vi "EC_Applied_Motion_RXRYRZ_20120124_3ch.vi"() -> ()   [LabVIEW 2014]
uses:
  <vilib>/Utility/file.llb/Read From Spreadsheet File (I64).vi
  <vilib>/Utility/file.llb/Read From Spreadsheet File (string).vi
  <vilib>/Instr/_visa.llb/VISA Configure Serial Port (Instr).vi
  <userlib>/caLab/Private/Put_DBL-1D_PV-1D.vi
  <vilib>/Utility/file.llb/Write To Spreadsheet File (I64).vi
  <vilib>/Utility/file.llb/Write To Spreadsheet File (string).vi
panel:
  out "Z Velocity MV mm/sec":dbl format="%.3f"
  out "Z Position MV mm":dbl
  out "Y Velocity MV mm/sec":dbl format="%.3f"
  out "Y Position MV mm":dbl
  out "X Velocity MV mm/sec":dbl format="%.3f"
  out "X Position MV mm":dbl
  out "Presets":i32[][](array[numeric])
  in  "stop":bool
  in  "Tab Control 3":enum32{"Status", "Reset"}(tab)
  out "Y in Range":bool
  out "Y Scan":bool
  out "Y in Motion":bool
  out "Y Backlash corr":bool
  out "X  in Range":bool
  out "X Scan":bool
  out "X  in Motion":bool
  out "X Backlash corr":bool
  out "Z in Range":bool
  out "Z Scan":bool
  out "Z in Motion":bool
  out "Z Backlash corr":bool
  out "X Ready":bool
  out "Y Ready":bool
  out "Z Ready":bool
  in  "Reset Y Position mm":dbl
  out "Reset Y Motor Steps":i32
  in  "Reset X Position mm":dbl
  out "Reset X Motor Steps":i32
  in  "Reset Z Position mm":dbl
  out "Reset Z Motor Steps":i32
  in  "Reset":bool
  in  "Tab Control 2":enum32{"mm", "step"}(tab)
  in  "X Scan Length SP mm":dbl
  in  "X Scan Velocity SP mm/sec":dbl
  in  "X Scan set":bool
  in  "Y Scan Length SP mm":dbl
  in  "Y Scan Velocity SP mm/sec":dbl
  in  "Y Scan set":bool
  in  "Z Scan Length SP mm":dbl
  in  "Z Scan Velocity SP mm/sec":dbl
  in  "Z Scan set":bool
  in  "X Scan Velocity SP steps/sec":i32=1 min=1 max=102400 step=1
  in  "X Scan Length SP steps":i32 min=-500000 max=500000 step=100
  out "X Scan length MV mm":dbl
  out "X Scan velocity MV mm/sec":dbl format="%#_6f"
  in  "Y Scan Velocity SP steps/sec":i32=1 min=1 max=102400 step=1
  in  "Y Scan Length SP steps":i32 min=-1000000 max=0 step=100
  out "Y Scan length MV mm":dbl
  out "Y Scan velocity MV mm/sec":dbl format="%#_6f"
  in  "Z Scan Velocity SP steps/sec":i32=1 min=1 max=102400 step=1
  in  "Z Scan Length SP steps":i32 min=-204724 max=102195276 step=100
  out "Z Scan length MV mm":dbl
  out "Z Scan velocity MV mm/sec":dbl format="%#_6f"
  out "atan Y/Z":dbl
  in  "Tab Control":enum32{"mm", "preset", "step"}(tab)
  in  "X Position SP mm":dbl
  in  "X Velocity SP mm/sec":dbl
  in  "X Move Set":bool
  in  "Y Move Set":bool
  in  "Y Position SP mm":dbl
  in  "Y Velocity SP mm/sec":dbl
  in  "Z Position SP mm":dbl
  in  "Z Velocity SP mm/sec":dbl
  in  "Z Move Set":bool
  in  "Add Button":bool
  in  "String":string
  in  "Delete Button":bool
  in  "Preset positions":i32(ring) items=["ZERO", "Default", "CDOSE", "QMS", "test", "test2", "test3"]
  in  "Set Button":bool
  in  "X Velocity SP step/sec":i32 min=1 max=50000
  in  "Y Velocity SP step/sec":i32 min=1 max=50000
  in  "Z Velocity SP step/sec":i32 min=1 max=5000
  in  "Y Step SP":i32=-20000 min=-800000 max=800000 step=500
  in  "X Step SP":i32=-20000 min=-750000 max=750000 step=500
  in  "Z Step SP":i32=-20000 min=-3000 max=102400000 step=500
  out "X Step PV":i32 max=2000
  out "Y Step PV":i32 max=2000
  out "Z Step PV":i32 max=2000
  out "R Step PV":i32 max=2000
  out "X Scan Duration":dbl
  out "Y Scan Duration":dbl
  out "Z Scan Duration":dbl
  out "Z COM PORT":refnum<visa-resource-name>="COM5"
  out "Z Backlash steps/sec":i32
  out "Z Backlash":i32
  out "Z Holding Current %":i32
  out "Z Run Current %":i32
  out "Z offset mm":dbl
  out "Z mm/rev":dbl
  out "Z steps/rev":u32
  out "Z  velocity PV step/sec":i32
  out "Z MINPOS":i32=-94296
  out "Z MAXPOS":i32=-34296
  in  "Z Scan OK":bool
  in  "Z Go":bool
  out "Z Position mm PV":dbl
  out "X Position mm PV":dbl
  out "X velocity PV step/sec":i32
  in  "X Scan OK":bool
  in  "X Go":bool
  out "X Backlash steps/sec":i32
  out "X Backlash":i32
  out "X Holding Current %":i32
  out "X Run Current %":i32
  out "X offset mm":dbl
  out "X mm/rev":dbl
  out "X steps/rev":u32
  out "X MAXPOS":i32=-34296
  out "X MINPOS":i32=-94296
  out "X COM PORT":refnum<visa-resource-name>="COM5"
  out "Y Backlash steps/sec":i32
  out "Y Backlash":i32
  out "Y Holding Current %":i32
  out "Y Run Current %":i32
  in  "Scan Cancel":bool
  out "Y Position mm PV":dbl
  out "Y offset mm":dbl
  out "Y mm/rev":dbl
  out "Y steps/rev":u32
  out "Y velocity PV step/sec":i32
  in  "Y Scan OK":bool
  in  "Scan Go":bool
  in  "Stop":bool
  in  "Y Go":bool
  out "Y MINPOS":i32=-94296
  out "Y MAXPOS":i32=-34296
  out "Y COM PORT":refnum<visa-resource-name>="COM5"
  # "REF"
  # "Current position"
  # "Goto position"
  # "RX"
  # "RX"
  # "RY"
  # "RY"
  # "RZ"
  # "RZ"
  # "21-22-23"
  # "R,L = green"
  # "COM21:COM22:COM23"
  # "L"
  # "M"
  # "B"
  # "S"
  # "R"
  # "Preset position"
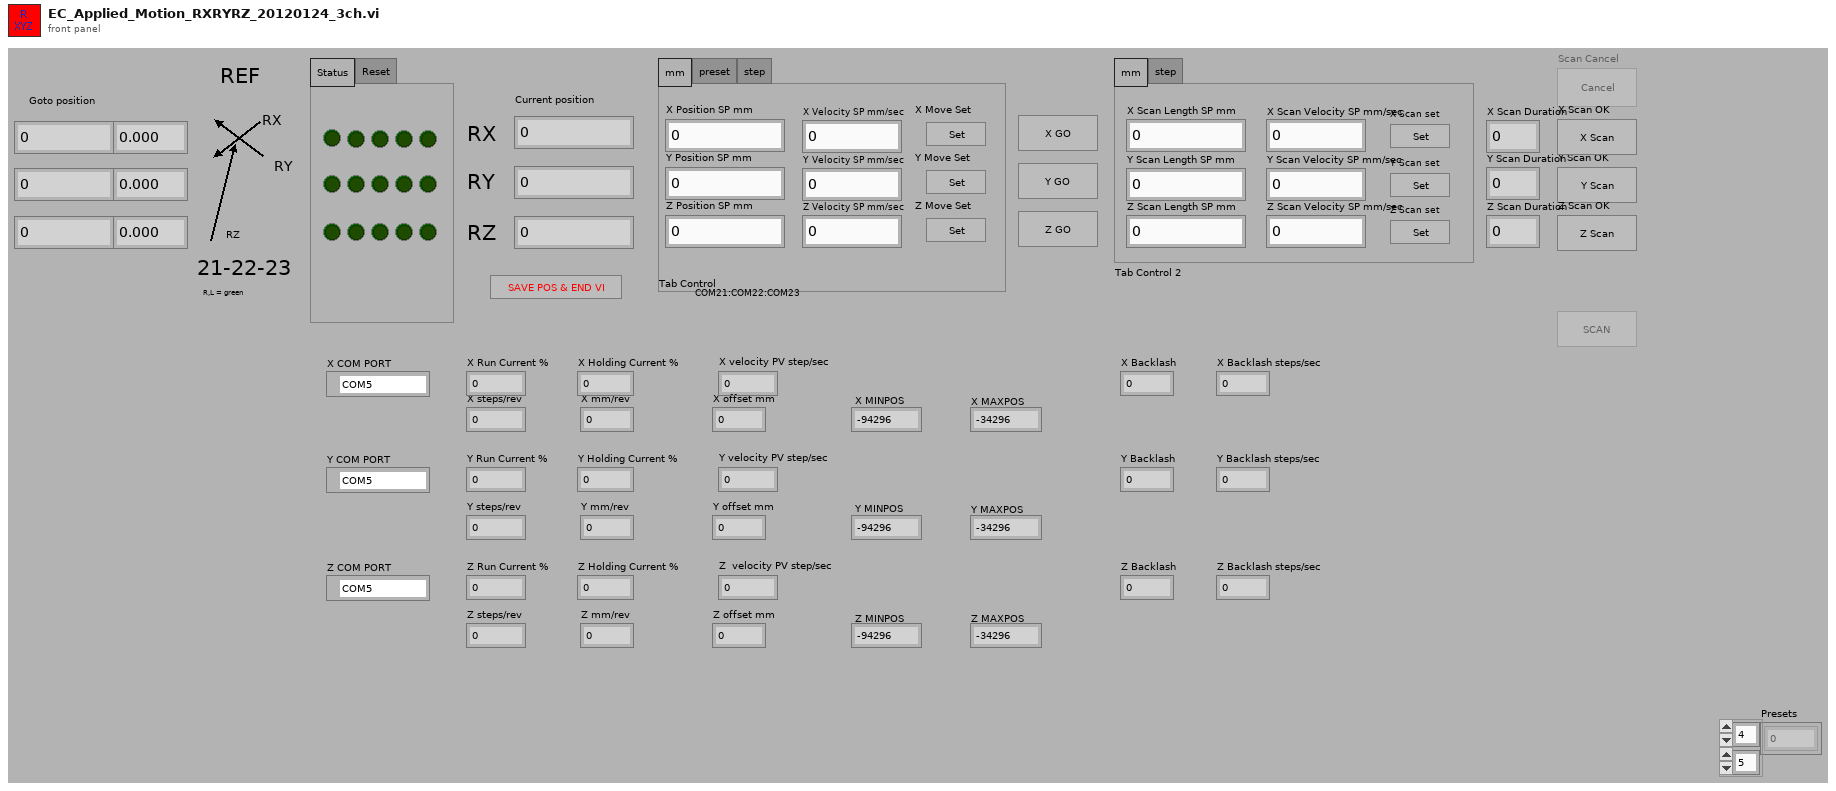
[diagram p1: front panel]
types:
  T1 = enum16{"Power-up Signature", "Accel Rate", "Accel Max", "Bit Rate", "Buffer Status", "Change Current", "Commence Jogging", "Change Jog Speed", "Continue", "Define Address", "Distance for FC,FM,FO,FY", "Decel Rate", "Distance or Position", "Define Limits", "Encoder Deadband", "Encoder Function", "Encoder Position", "Encoder Ratio", "Feed to Length with Speed Change", "Feed to Length", "Feed to Sensor with Mask Dist", "Feed to Length & Set Output", "Feed to Position", "Feed to Sensor", "Feed to Sensor w/safety", "Follow Handwheel", "Immediate Distance?", "Immediate Encoder?", "Immediate Low Output", "Immediate High Output", "Immediate Position?", "Input Status?", "Jog Accel/Decel", "Jog Disable", "Jog Enable", "Jog Speed", "Motor Disable", "Motor Enable", "Microstep Resolution", "Power up Current", "Power up Mode", "Pause", "Request Status", "Revision Level?", "Seek Home", "Stop Jogging", "Stop & Kill Buffer", "Set Output", "Set ABS Position", "Send String", "Stop", "Velocity for Speed Change", "Velocity Setting", "Wait for Input", "Wait Time"}
  T2 = enum8{"Enabled", "Disabled", "Disabled and Grayed Out"}
  T3 = cluster{"first row[0]":i64, "first row[1]":i64, "first row[2]":i64, "first row[3]":i64, "first row[4]":i64, "first row[5]":i64, "first row[6]":i64, "first row[7]":i64, "first row[8]":i64}
  T4 = cluster{"Value[0]":i32, "Value[1]":i32, "Value[2]":i32, "Value[3]":i32, "Value[4]":i32, "Value[5]":i32, "Value[6]":i32, "Value[7]":i32, "Value[8]":i32}
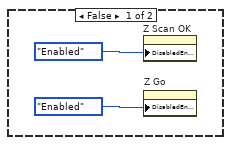
[diagram p5: hidden frame]
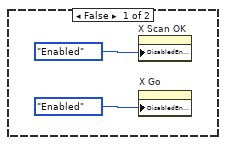
[diagram p8: hidden frame]
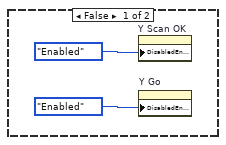
[diagram p11: hidden frame]
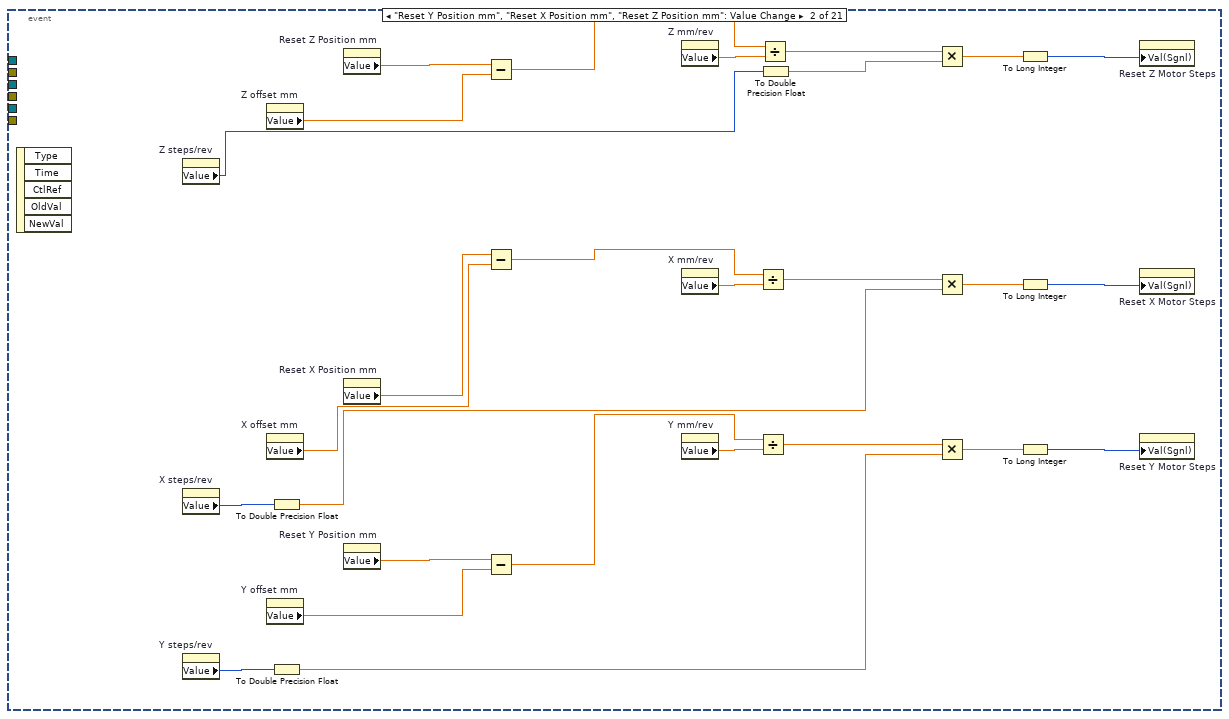
[diagram p14: hidden frame]
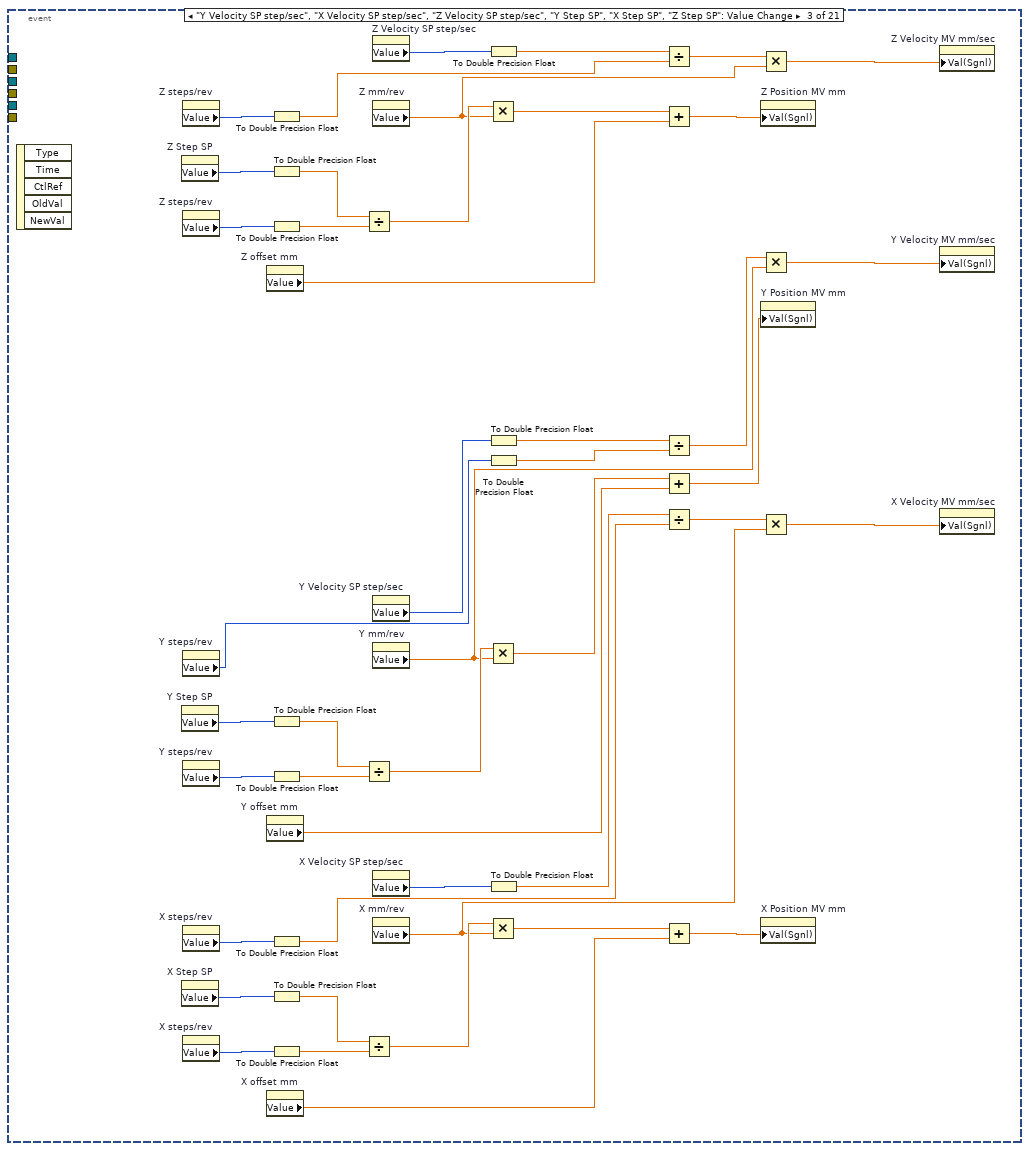
[diagram p15: hidden frame]
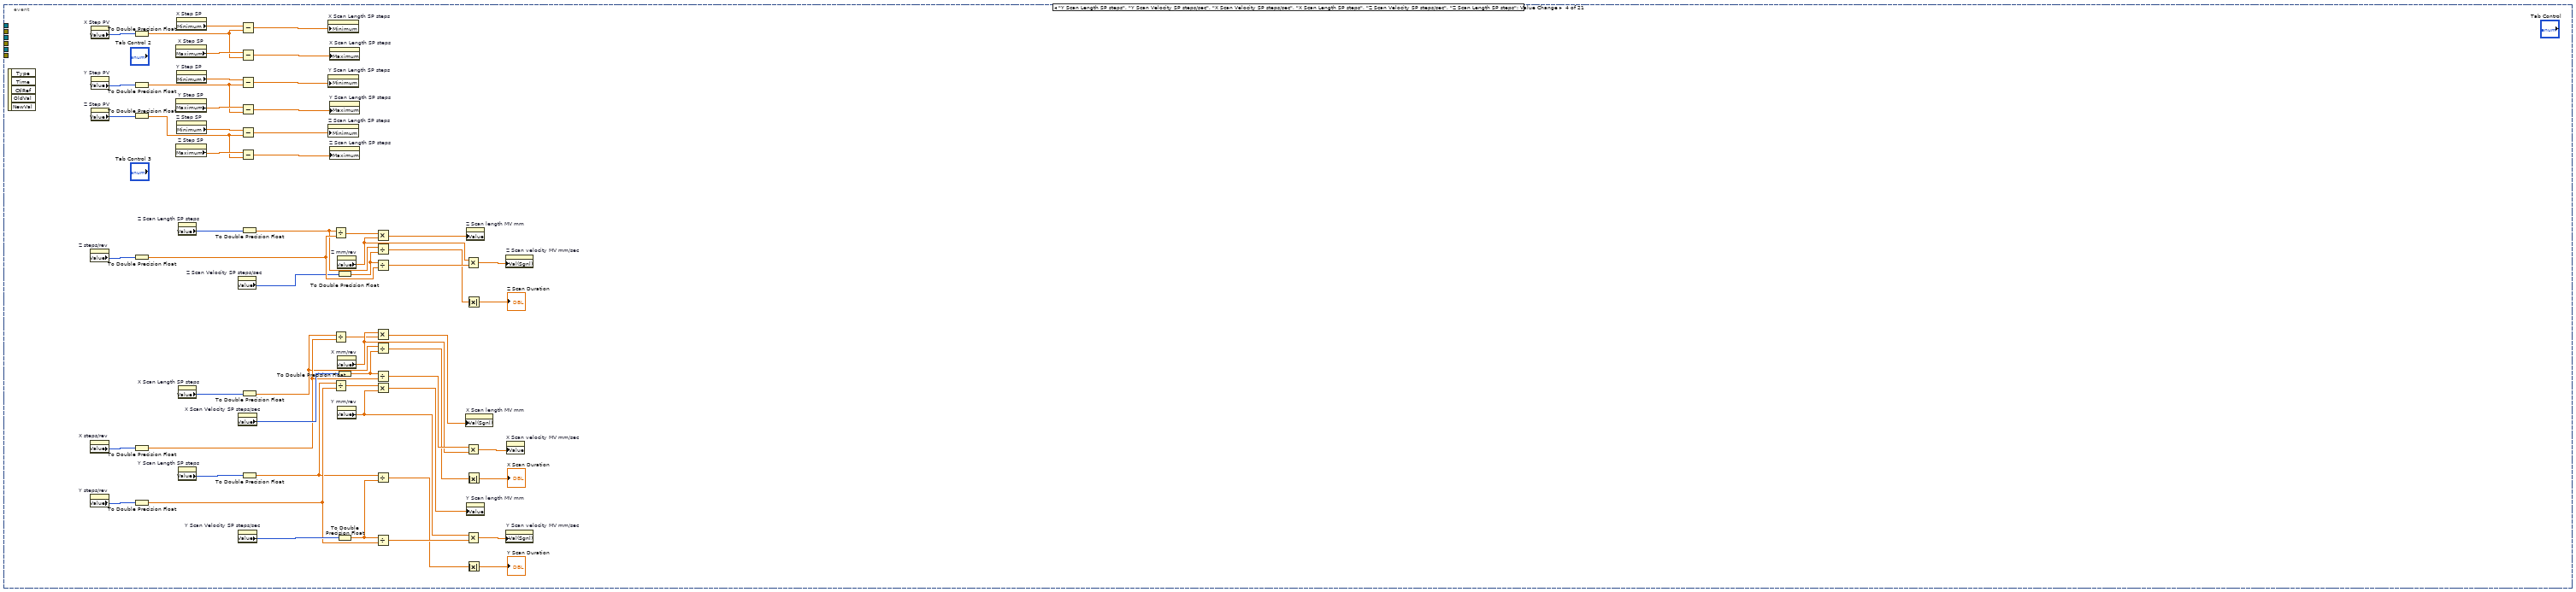
[diagram p16: hidden frame]
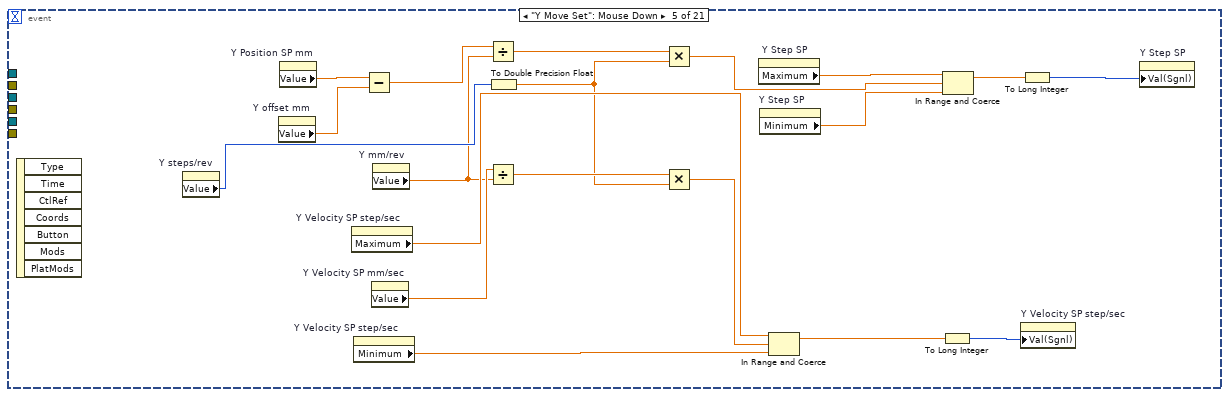
[diagram p17: hidden frame]
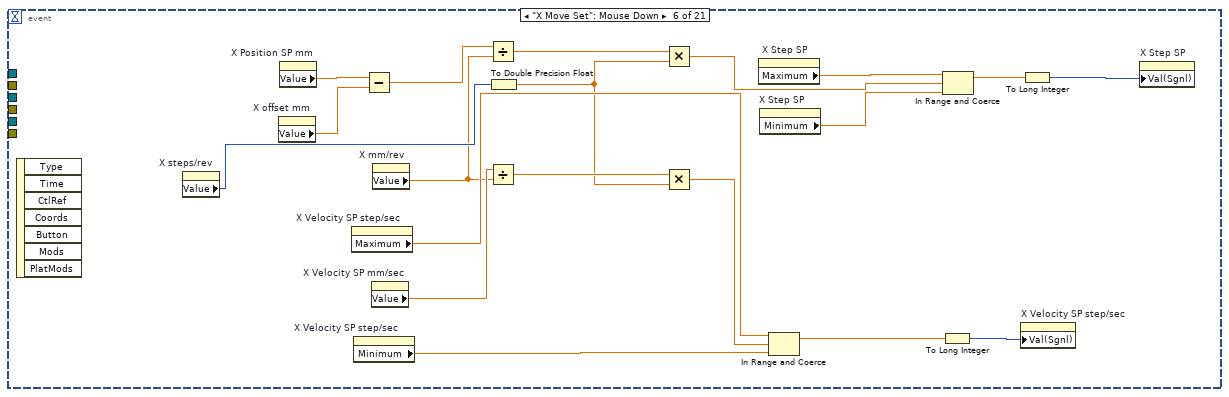
[diagram p18: hidden frame]
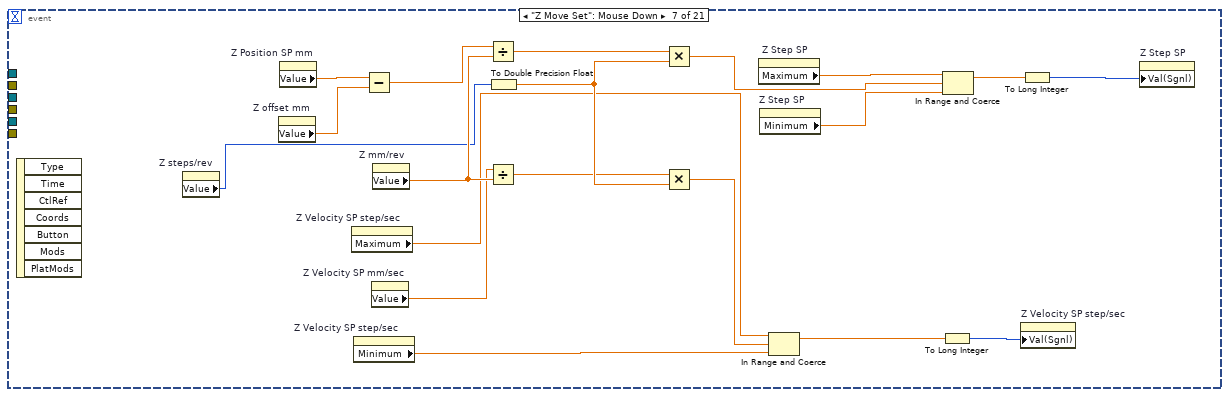
[diagram p19: hidden frame]
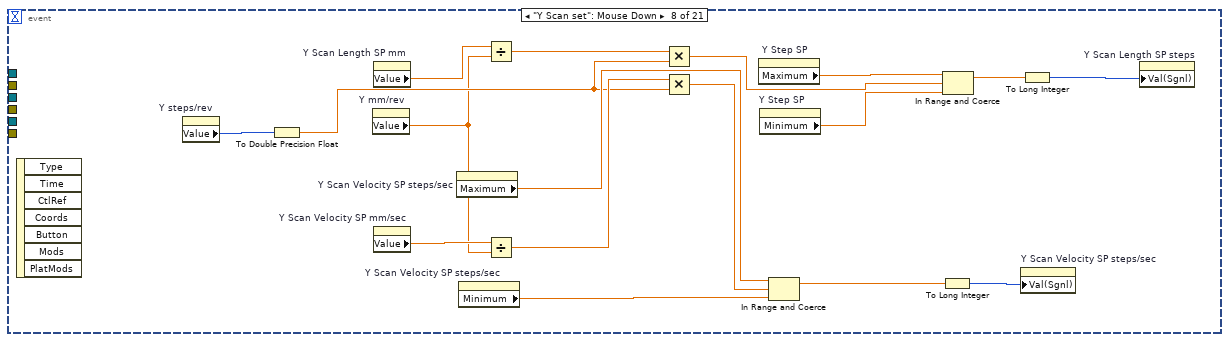
[diagram p20: hidden frame]
diagram:
  (unwired) FALSE
  w19 = 0 ("dimension size")
  n1 = flat-sequence {
    tunnel: [w78] -> w5
    tunnel: [w77] -> w4
    tunnel: w5 -> [w92]
    tunnel: w4 -> [w91]
    tunnel: [w90] -> w3
    tunnel: [w89] -> w2
    tunnel: [w100] -> w49
    tunnel: [w99] -> w48
    tunnel: w3 -> [w102]
    tunnel: w2 -> [w101]
    tunnel: w49 -> [w117]
    tunnel: w48 -> [w116]
    tunnel: [w118] -> w47
    tunnel: [w119] -> w46
    tunnel: [w120] -> w1
    tunnel: [w131] -> w44
    tunnel: [w132] -> w45
    tunnel: w47 -> [w132]
    tunnel: w46 -> [w131]
    tunnel: w1 -> [w129]
    frame #0 {
      "Z Run Current %" <- 100 ("Z Run Current %")
      "Z Holding Current %" <- 50 ("Z Holding Current %")
    }
    frame #1 {
      "Z Backlash steps/sec" <- 1000 ("Z Backlash steps/sec")
      "Z Backlash" <- -2500 ("Z Backlash")
    }
    frame #2 {
      w68 = 2.54 ("Z mm/rev")
      w67 = u32 20000 ("step/rev")
      w69 = 5000 ("Value (Signaling)")
      n2 = property on="Z Velocity SP step/sec" class="DigNum (strict)"("Minimum"=1.0 ("Data Entry Limits:Minimum")) -> ()  [unwired: 2 in, 2 out]
      n3 = property on="Z Scan Velocity SP mm/sec" class="DigNum (strict)"("Val(Sgnl)"=0.1 ("Value (Signaling)")) -> ()  [unwired: 2 in, 2 out]
      n4 = property on="Z Velocity SP step/sec" class="DigNum (strict)"("Val(Sgnl)"=w69) -> ()  [unwired: 2 in, 2 out]
      n5 = To Double Precision Float(number=w69) -> (double precision float=w73:dbl)
      n6 = property on="Z Velocity SP step/sec" class="DigNum (strict)"("Maximum"=w73) -> ()  [unwired: 2 in, 2 out]
      n7 = To Double Precision Float(number=w67) -> (double precision float=w72:dbl)
      n8 = Divide(x=w73, y=w72) -> (x/y=w70:dbl)
      n9 = Multiply(x=w70, y=w68) -> (x*y=w71:dbl)
      n10 = property on="Z Velocity SP mm/sec" class="DigNum (strict)"("Val(Sgnl)"=w71) -> ()  [unwired: 2 in, 2 out]
      "Z mm/rev" <- w68
      "Z steps/rev" <- w67
    }
    frame #3 {
      w75 = -3000 ("lower limit")
      w74 = 102400000 ("upper limit")
      n11 = property on="Z Step SP" class="DigNum (strict)"("Minimum"=w75) -> ()  [unwired: 2 in, 2 out]
      n12 = property on="Z Step SP" class="DigNum (strict)"("Maximum"=w74) -> ()  [unwired: 2 in, 2 out]
      "Z offset mm" <- 0.0 ("Z offset mm")
      "Z MINPOS" <- w75
      "Z MAXPOS" <- w74
    }
    frame #4 {
      w85 = refnum<visa-resource-name> "COM23" ("COM PORT")
      w83 = u16 0 items=["None", "XON/XOFF", "RTS/CTS", "XON/XOFF & RTS/CTS", "DTR/DSR", "XON/XOFF & DTR/DSR"] ("flow control (0:none)")
      w82 = u16 10 items=["1.0"=10, "1.5"=15, "2.0"=20] ("stop bits (10: 1 bit)")
      # "Stop bits"
      n13 = call-poly "VISA Configure Serial Port"("VISA resource name"=w85, "timeout (10sec)"=u32 10000, "baud rate (9600)"=u32 9600, "data bits (8)"=u16 8, "parity (0:none)"=enum16{"None", "Odd", "Even", "Mark", "Space"}."None", "stop bits (10: 1 bit)"=w82, "flow control (0:none)"=w83) -> ("VISA resource name out"=w78:refnum<visa-resource-name>, "error out"=w77:errorcluster)  [unwired: 7 in]
      "Z COM PORT" <- w85
    }
    frame #5 {
      # "Run Current %"
      n14 = property on="Z Run Current %" class="DigNum (strict)"() -> ("Value"=w93:i32)  [unwired: 2 in, 2 out]
      n15 = Divide(x=w93, y=100) -> (x/y=w94:dbl)
      n16 = Multiply(x=w94, y=3.5) -> (x*y=w88:dbl)
      n17 = Number To Fractional String(number=w88) -> (F-format string=w95:string)  [unwired: 3 in]
      n18 = call "Applied Send Command.vi"("error in (no error)"=w91, "Extra"=w95, "Command"=T1."Change Current", "VISA resource name"=w92) -> ("error out"=w89:errorcluster, "VISA resource name out"=w90:refnum<visa-resource-name>)  [unwired: 3 in, 1 out]
    }
    frame #6 {
      # "VELOCITY"
      n19 = property on="Z steps/rev" class="DigNum (strict)"() -> ("Value"=w98:u32)  [unwired: 2 in, 2 out]
      n20 = property on="Z Velocity SP step/sec" class="DigNum (strict)"() -> ("Value"=w97:i32)  [unwired: 2 in, 2 out]
      n21 = Divide(x=w97, y=w98) -> (x/y=w105:dbl)
      n22 = Number To Fractional String(number=w105) -> (F-format string=w107:string)  [unwired: 3 in]
      n23 = call "Applied Send Command.vi"("error in (no error)"=w101, "Extra"=w107, "Command"=T1."Velocity Setting", "VISA resource name"=w102) -> ("error out"=w108:errorcluster, "VISA resource name out"=w115:refnum<visa-resource-name>)  [unwired: 3 in, 1 out]
      n24 = call "Time Delay2"("error in (no error)"=w108, "Delay Time (s)"=0.1) -> ("error out"=w113:errorcluster)  [unwired: 9 in]
      n25 = call "Applied Send Command.vi"("error in (no error)"=w113, "Extra"="", "Command"=T1."Velocity Setting", "VISA resource name"=w115) -> ("error out"=w99:errorcluster, "read buffer"=w111:string, "VISA resource name out"=w100:refnum<visa-resource-name>)  [unwired: 3 in]
      n26 = Fract/Exp String To Number(string=w111, offset=3) -> (number=w106:dbl)  [unwired: 2 in, 1 out]
      n27 = Multiply(x=w106, y=w98) -> (x*y=w103:dbl)
      n28 = property on="Z  velocity PV step/sec" class="DigNum (strict)"("Val(Sgnl)"=w103) -> ()  [unwired: 2 in, 2 out]
    }
    frame #7 {
      # "GET CURRENT POSITION"
      n29 = call "Applied Send Command.vi"("error in (no error)"=w116, "Extra"="", "Command"=T1."Immediate Position?", "VISA resource name"=w117) -> ("error out"=w122:errorcluster, "read buffer"=w124:string, "VISA resource name out"=w118:refnum<visa-resource-name>)  [unwired: 3 in]
      n30 = call "Time Delay8"("error in (no error)"=w122, "Delay Time (s)"=0.1) -> ("error out"=w119:errorcluster)  [unwired: 9 in]
      n31 = Hexadecimal String To Number(string=w124, offset=3) -> (number=w120:u32)  [unwired: 1 in, 1 out]
    }
    frame #8 {
      n32 = property on="Z Step SP" class="DigNum (strict)"() -> ("Maximum"=w128:dbl)  [unwired: 2 in, 2 out]
      n33 = property on="Z Step SP" class="DigNum (strict)"() -> ("Minimum"=w127:dbl)  [unwired: 2 in, 2 out]
      n34 = property on="Z Step SP" class="DigNum (strict)"("Val(Sgnl)"=w129) -> ()  [unwired: 2 in, 2 out]
      n35 = In Range and Coerce(upper limit=w128, x=w129, lower limit=w127) -> (In Range?=w130:bool)  [unwired: 1 out]
      n36 = property on="Z in Range" class="Bool (strict)"("Val(Sgnl)"=w130) -> ()  [unwired: 2 in, 2 out]
    }
  }
  n37 = flat-sequence {
    frame #0 {
      n38 = property on="X Scan" class="Bool (strict)"("Val(Sgnl)"=FALSE ("Value (Signaling)")) -> ()  [unwired: 2 in, 2 out]
      n39 = property on="Y Scan" class="Bool (strict)"("Val(Sgnl)"=FALSE ("Value (Signaling)")) -> ()  [unwired: 2 in, 2 out]
      n40 = property on="Z Scan" class="Bool (strict)"("Val(Sgnl)"=FALSE ("Value (Signaling)")) -> ()  [unwired: 2 in, 2 out]
      n41 = property on="Scan Go" class="Bool"("DisabledEnum"=T2."Disabled and Grayed Out" ("Disabled")) -> ()  [unwired: 2 in, 2 out]
      n42 = property on="Scan Cancel" class="Bool"("DisabledEnum"=T2."Disabled and Grayed Out" ("Disabled")) -> ()  [unwired: 2 in, 2 out]
    }
    frame #1 {
      n43 = property on="Y Backlash corr" class="Bool (strict)"("Val(Sgnl)"=FALSE ("Value (Signaling)")) -> ()  [unwired: 2 in, 2 out]
      n44 = property on="X Backlash corr" class="Bool (strict)"("Val(Sgnl)"=FALSE ("Value (Signaling)")) -> ()  [unwired: 2 in, 2 out]
      n45 = property on="Z Backlash corr" class="Bool (strict)"("Val(Sgnl)"=FALSE ("Value (Signaling)")) -> ()  [unwired: 2 in, 2 out]
    }
  }
  n46 = flat-sequence {
    tunnel: [w158] -> w13
    tunnel: [w157] -> w12
    tunnel: w13 -> [w172]
    tunnel: w12 -> [w171]
    tunnel: [w170] -> w11
    tunnel: [w169] -> w10
    tunnel: w11 -> [w180]
    tunnel: w10 -> [w179]
    tunnel: [w178] -> w9
    tunnel: [w177] -> w8
    tunnel: [w197] -> w53
    tunnel: w9 -> [w200]
    tunnel: w8 -> [w199]
    tunnel: [w198] -> w7
    tunnel: [w196] -> w6
    tunnel: [w209] -> w59
    tunnel: [w212] -> w60
    tunnel: w53 -> [w209]
    tunnel: w7 -> [w212]
    tunnel: w6 -> [w210]
    frame #0 {
      "Y Run Current %" <- 100 ("Run Current %")
      "Y Holding Current %" <- 50 ("Holding Current %")
    }
    frame #1 {
      "Y Backlash" <- 5000 ("Backlash2")
      "Y Backlash steps/sec" <- 10000 ("Value (Signaling)")
    }
    frame #2 {
      w148 = 0.21167 ("MM/rev")
      w151 = u32 20000 ("step/rev")
      w146 = 50000 ("Value (Signaling)")
      n47 = property on="Y Velocity SP step/sec" class="DigNum (strict)"("Minimum"=1.0 ("Data Entry Limits:Minimum")) -> ()  [unwired: 2 in, 2 out]
      n48 = property on="Y Scan Velocity SP mm/sec" class="DigNum (strict)"("Val(Sgnl)"=0.1 ("Value (Signaling)")) -> ()  [unwired: 2 in, 2 out]
      n49 = property on="Y Velocity SP step/sec" class="DigNum (strict)"("Val(Sgnl)"=w146) -> ()  [unwired: 2 in, 2 out]
      n50 = To Double Precision Float(number=w146) -> (double precision float=w152:dbl)
      n51 = property on="Y Velocity SP step/sec" class="DigNum (strict)"("Maximum"=w152) -> ()  [unwired: 2 in, 2 out]
      n52 = To Double Precision Float(number=w151) -> (double precision float=w150:dbl)
      n53 = Divide(x=w152, y=w150) -> (x/y=w147:dbl)
      n54 = Multiply(x=w147, y=w148) -> (x*y=w149:dbl)
      n55 = property on="Y Velocity SP mm/sec" class="DigNum (strict)"("Val(Sgnl)"=w149) -> ()  [unwired: 2 in, 2 out]
      "Y steps/rev" <- w151
      "Y mm/rev" <- w148
    }
    frame #3 {
      w155 = -800000 ("lower limit")
      w156 = 800000 ("upper limit")
      n56 = property on="Y Step SP" class="DigNum (strict)"("Minimum"=w155) -> ()  [unwired: 2 in, 2 out]
      n57 = property on="Y Step SP" class="DigNum (strict)"("Maximum"=w156) -> ()  [unwired: 2 in, 2 out]
      "Y MAXPOS" <- w156
      "Y MINPOS" <- w155
      "Y offset mm" <- 0.0 ("offset")
    }
    frame #4 {
      w165 = refnum<visa-resource-name> "COM22" ("COM PORT")
      w163 = u16 0 items=["None", "XON/XOFF", "RTS/CTS", "XON/XOFF & RTS/CTS", "DTR/DSR", "XON/XOFF & DTR/DSR"] ("flow control (0:none)")
      w162 = u16 10 items=["1.0"=10, "1.5"=15, "2.0"=20] ("stop bits (10: 1 bit)")
      # "Stop bits"
      n58 = call-poly "VISA Configure Serial Port"("VISA resource name"=w165, "timeout (10sec)"=u32 10000, "baud rate (9600)"=u32 9600, "data bits (8)"=u16 8, "parity (0:none)"=enum16{"None", "Odd", "Even", "Mark", "Space"}."None", "stop bits (10: 1 bit)"=w162, "flow control (0:none)"=w163) -> ("VISA resource name out"=w158:refnum<visa-resource-name>, "error out"=w157:errorcluster)  [unwired: 7 in]
      "Y COM PORT" <- w165
    }
    frame #5 {
      n59 = property on="Y Run Current %" class="DigNum (strict)"() -> ("Value"=w173:i32)  [unwired: 2 in, 2 out]
      n60 = Divide(x=w173, y=100) -> (x/y=w174:dbl)
      n61 = Multiply(x=w174, y=3.5) -> (x*y=w168:dbl)
      n62 = Number To Fractional String(number=w168) -> (F-format string=w175:string)  [unwired: 3 in]
      n63 = call "Applied Send Command.vi"("error in (no error)"=w171, "Extra"=w175, "Command"=T1."Change Current", "VISA resource name"=w172) -> ("error out"=w169:errorcluster, "VISA resource name out"=w170:refnum<visa-resource-name>)  [unwired: 3 in, 1 out]
    }
    frame #6 {
      # "VELOCITY"
      n64 = property on="Y steps/rev" class="DigNum (strict)"() -> ("Value"=w184:u32)  [unwired: 2 in, 2 out]
      n65 = property on="Y Velocity SP step/sec" class="DigNum (strict)"() -> ("Value"=w181:i32)  [unwired: 2 in, 2 out]
      n66 = Divide(x=w181, y=w184) -> (x/y=w183:dbl)
      n67 = Number To Fractional String(number=w183) -> (F-format string=w187:string)  [unwired: 3 in]
      n68 = call "Applied Send Command.vi"("error in (no error)"=w179, "Extra"=w187, "Command"=T1."Velocity Setting", "VISA resource name"=w180) -> ("error out"=w188:errorcluster, "VISA resource name out"=w195:refnum<visa-resource-name>)  [unwired: 3 in, 1 out]
      n69 = call "Time Delay36"("error in (no error)"=w188, "Delay Time (s)"=0.1) -> ("error out"=w193:errorcluster)  [unwired: 9 in]
      n70 = call "Applied Send Command.vi"("error in (no error)"=w193, "Extra"="", "Command"=T1."Velocity Setting", "VISA resource name"=w195) -> ("error out"=w177:errorcluster, "read buffer"=w191:string, "VISA resource name out"=w178:refnum<visa-resource-name>)  [unwired: 3 in]
      n71 = Fract/Exp String To Number(string=w191, offset=3) -> (number=w186:dbl)  [unwired: 2 in, 1 out]
      n72 = Multiply(x=w186, y=w184) -> (x*y=w185:dbl)
      n73 = property on="Y velocity PV step/sec" class="DigNum (strict)"("Val(Sgnl)"=w185) -> ()  [unwired: 2 in, 2 out]
    }
    frame #7 {
      # "GET CURRENT POSITION"
      n74 = call "Applied Send Command.vi"("error in (no error)"=w199, "Extra"="", "Command"=T1."Immediate Position?", "VISA resource name"=w200) -> ("error out"=w202:errorcluster, "read buffer"=w204:string, "VISA resource name out"=w198:refnum<visa-resource-name>)  [unwired: 3 in]
      n75 = call "Time Delay37"("error in (no error)"=w202, "Delay Time (s)"=0.1) -> ("error out"=w197:errorcluster)  [unwired: 9 in]
      n76 = Hexadecimal String To Number(string=w204, offset=3) -> (number=w196:u32)  [unwired: 1 in, 1 out]
    }
    frame #8 {
      n77 = property on="Y Step SP" class="DigNum (strict)"() -> ("Maximum"=w208:dbl)  [unwired: 2 in, 2 out]
      n78 = property on="Y Step SP" class="DigNum (strict)"() -> ("Minimum"=w207:dbl)  [unwired: 2 in, 2 out]
      n79 = property on="Y Step SP" class="DigNum (strict)"("Val(Sgnl)"=w210) -> ()  [unwired: 2 in, 2 out]
      n80 = In Range and Coerce(upper limit=w208, x=w210, lower limit=w207) -> (In Range?=w211:bool)  [unwired: 1 out]
      n81 = property on="Y in Range" class="Bool (strict)"("Val(Sgnl)"=w211) -> ()  [unwired: 2 in, 2 out]
    }
  }
  n82 = flat-sequence {
    tunnel: [w230] -> w18
    tunnel: [w229] -> w17
    tunnel: w18 -> [w247]
    tunnel: w17 -> [w246]
    tunnel: [w245] -> w16
    tunnel: [w244] -> w15
    tunnel: [w250] -> w58
    tunnel: w16 -> [w258]
    tunnel: w15 -> [w257]
    tunnel: [w251] -> w14
    tunnel: w58 -> [w272]
    tunnel: [w271] -> w52
    tunnel: [w269] -> w51
    tunnel: [w274] -> w50
    tunnel: w14 -> [w273]
    tunnel: [w283] -> w56
    tunnel: [w284] -> w57
    tunnel: w52 -> [w284]
    tunnel: w51 -> [w283]
    tunnel: w50 -> [w279]
    frame #0 {
      "X Run Current %" <- 100 ("Run Current %")
      "X Holding Current %" <- 50 ("Holding Current %")
    }
    frame #1 {
      "X Backlash steps/sec" <- 10000 ("Value (Signaling)")
      "X Backlash" <- 5000 ("Backlash2")
    }
    frame #2 {
      w219 = 0.21167 ("MM/rev")
      w222 = u32 20000 ("step/rev")
      w217 = 50000 ("Value (Signaling)")
      n83 = property on="X Velocity SP step/sec" class="DigNum (strict)"("Minimum"=1.0 ("Data Entry Limits:Minimum")) -> ()  [unwired: 2 in, 2 out]
      n84 = property on="X Velocity SP step/sec" class="DigNum (strict)"("Val(Sgnl)"=w217) -> ()  [unwired: 2 in, 2 out]
      n85 = property on="X Scan Velocity SP mm/sec" class="DigNum (strict)"("Val(Sgnl)"=0.1 ("Value (Signaling)")) -> ()  [unwired: 2 in, 2 out]
      n86 = To Double Precision Float(number=w217) -> (double precision float=w223:dbl)
      n87 = property on="X Velocity SP step/sec" class="DigNum (strict)"("Maximum"=w223) -> ()  [unwired: 2 in, 2 out]
      n88 = To Double Precision Float(number=w222) -> (double precision float=w221:dbl)
      n89 = Divide(x=w223, y=w221) -> (x/y=w218:dbl)
      n90 = Multiply(x=w218, y=w219) -> (x*y=w220:dbl)
      n91 = property on="X Velocity SP mm/sec" class="DigNum (strict)"("Val(Sgnl)"=w220) -> ()  [unwired: 2 in, 2 out]
      "X steps/rev" <- w222
      "X mm/rev" <- w219
    }
    frame #3 {
      w228 = -750000 ("lower limit")
      w227 = 750000 ("upper limit")
      n92 = property on="X Step SP" class="DigNum (strict)"("Minimum"=w228) -> ()  [unwired: 2 in, 2 out]
      n93 = property on="X Step SP" class="DigNum (strict)"("Maximum"=w227) -> ()  [unwired: 2 in, 2 out]
      "X offset mm" <- 0.0 ("offset")
      "X MAXPOS" <- w227
      "X MINPOS" <- w228
    }
    frame #4 {
      w237 = refnum<visa-resource-name> "COM21" ("COM PORT")
      w235 = u16 0 items=["None", "XON/XOFF", "RTS/CTS", "XON/XOFF & RTS/CTS", "DTR/DSR", "XON/XOFF & DTR/DSR"] ("flow control (0:none)")
      w234 = u16 10 items=["1.0"=10, "1.5"=15, "2.0"=20] ("stop bits (10: 1 bit)")
      # "Stop bits"
      n94 = call-poly "VISA Configure Serial Port"("VISA resource name"=w237, "timeout (10sec)"=u32 10000, "baud rate (9600)"=u32 9600, "data bits (8)"=u16 8, "parity (0:none)"=enum16{"None", "Odd", "Even", "Mark", "Space"}."None", "stop bits (10: 1 bit)"=w234, "flow control (0:none)"=w235) -> ("VISA resource name out"=w230:refnum<visa-resource-name>, "error out"=w229:errorcluster)  [unwired: 7 in]
      "X COM PORT" <- w237
    }
    frame #5 {
      n95 = property on="X Run Current" class="DigNum (strict)"() -> ("Value"=w242:i32)  [unwired: 2 in, 2 out]
      n96 = Divide(x=w242, y=100) -> (x/y=w239:dbl)
      n97 = Multiply(x=3.5 ("y"), y=w239) -> (x*y=w241:dbl)
      n98 = Number To Fractional String(number=w241) -> (F-format string=w243:string)  [unwired: 3 in]
      n99 = call "Applied Send Command.vi"("error in (no error)"=w246, "Extra"=w243, "Command"=T1."Change Current", "VISA resource name"=w247) -> ("error out"=w245:errorcluster, "VISA resource name out"=w244:refnum<visa-resource-name>)  [unwired: 3 in, 1 out]
    }
    frame #6 {
      # "VELOCITY"
      n100 = property on="X steps/rev" class="DigNum (strict)"() -> ("Value"=w253:u32)  [unwired: 2 in, 2 out]
      n101 = property on="X Velocity SP step/sec" class="DigNum (strict)"() -> ("Value"=w254:i32)  [unwired: 2 in, 2 out]
      n102 = Divide(x=w254, y=w253) -> (x/y=w252:dbl)
      n103 = Number To Fractional String(number=w252) -> (F-format string=w259:string)  [unwired: 3 in]
      n104 = call "Applied Send Command.vi"("error in (no error)"=w258, "Extra"=w259, "Command"=T1."Velocity Setting", "VISA resource name"=w257) -> ("error out"=w260:errorcluster, "VISA resource name out"=w267:refnum<visa-resource-name>)  [unwired: 3 in, 1 out]
      n105 = call "Time Delay30"("error in (no error)"=w260, "Delay Time (s)"=0.1) -> ("error out"=w265:errorcluster)  [unwired: 9 in]
      n106 = call "Applied Send Command.vi"("error in (no error)"=w265, "Extra"="", "Command"=T1."Velocity Setting", "VISA resource name"=w267) -> ("error out"=w250:errorcluster, "read buffer"=w263:string, "VISA resource name out"=w251:refnum<visa-resource-name>)  [unwired: 3 in]
      n107 = Fract/Exp String To Number(string=w263, offset=3) -> (number=w256:dbl)  [unwired: 2 in, 1 out]
      n108 = Multiply(x=w256, y=w253) -> (x*y=w255:dbl)
      n109 = property on="X velocity PV step/sec" class="DigNum (strict)"("Val(Sgnl)"=w255) -> ()  [unwired: 2 in, 2 out]
    }
    frame #7 {
      # "GET CURRENT POSITION"
      n110 = call "Applied Send Command.vi"("error in (no error)"=w272, "Extra"="", "Command"=T1."Immediate Position?", "VISA resource name"=w273) -> ("error out"=w270:errorcluster, "read buffer"=w276:string, "VISA resource name out"=w271:refnum<visa-resource-name>)  [unwired: 3 in]
      n111 = call "Time Delay13"("error in (no error)"=w270, "Delay Time (s)"=0.1) -> ("error out"=w269:errorcluster)  [unwired: 9 in]
      n112 = Hexadecimal String To Number(string=w276, offset=3) -> (number=w274:u32)  [unwired: 1 in, 1 out]
    }
    frame #8 {
      n113 = property on="X Step SP" class="DigNum (strict)"() -> ("Maximum"=w282:dbl)  [unwired: 2 in, 2 out]
      n114 = property on="X Step SP" class="DigNum (strict)"() -> ("Minimum"=w281:dbl)  [unwired: 2 in, 2 out]
      n115 = property on="X Step SP" class="DigNum (strict)"("Val(Sgnl)"=w279) -> ()  [unwired: 2 in, 2 out]
      n116 = In Range and Coerce(upper limit=w282, x=w279, lower limit=w281) -> (In Range?=w280:bool)  [unwired: 1 out]
      n117 = property on="X  in Range" class="Bool (strict)"("Val(Sgnl)"=w280) -> ()  [unwired: 2 in, 2 out]
    }
  }
  n118 = call-poly <vilib>:"Read From Spreadsheet File.vi"("file path (dialog if empty)"=path "S:/SSE/SCL2/POS.TXT") -> ("first row"=w36:i64[])  [unwired: 6 in, 4 out]
  n119 = call-poly <vilib>:"Read From Spreadsheet File.vi"("file path (dialog if empty)"=path "S:/SSE/SCL2/PRESET.TXT") -> ("all rows"=w25:string[][])  [unwired: 6 in, 4 out]
  n120 = Array To Cluster(array=w36) -> (cluster=w35:T3)
  n121 = Transpose 2D Array(2D array=w25) -> (transposed array=w26:string[][])
  n122 = Unbundle(w35) -> ("first row[0]"=w33:i64, "first row[1]"=w32:i64, "first row[2]"=w31:i64)  [unwired: 6 out]
  n123 = Delete From Array(array=w26, index (row)=0) -> (deleted portion=w27:string[], array with subset deleted=w29:string[][])  [unwired: 2 in]
  n124 = property on="Reset X Motor Steps" class="DigNum (strict)"("Val(Sgnl)"=w33) -> ()  [unwired: 2 in, 2 out]
  n125 = property on="Reset Y Motor Steps" class="DigNum (strict)"("Val(Sgnl)"=w32) -> ()  [unwired: 2 in, 2 out]
  n126 = property on="Reset Z Motor Steps" class="DigNum (strict)"("Val(Sgnl)"=w31) -> ()  [unwired: 2 in, 2 out]
  n127 = property on="Preset positions" class="Ring (strict)"("Strings []"=w27) -> ()  [unwired: 2 in, 2 out]
  n128 = Transpose 2D Array(2D array=w29) -> (transposed array=w30:string[][])
  n129 = Decimal String To Number(string=w30) -> (number=w28:i32[][])  [unwired: 2 in, 1 out]
  n130 = Initialize Array(w19, w19, 4 ("dimension size")) -> (w22:i32[][])
  n131 = Build Array (concatenate)(w22, w28) -> (→"Presets":i32[][])
  n132 = while {
    tunnel: w60 -> [w306]
    tunnel: w59 -> [w309]
    tunnel: [w310] -> w40
    tunnel: [w308] -> w41
    tunnel: w57 -> [w305]
    tunnel: w56 -> [w304]
    tunnel: [w303] -> w55
    tunnel: [w302] -> w54
    tunnel: w45 -> [w301]
    tunnel: w44 -> [w300]
    tunnel: [w299] -> w43
    tunnel: [w298] -> w42
    tunnel: [w297] -> _
    tunnel: [w296] -> _
    stop <- "stop" stop-if-true
    n133 = flat-sequence {
      frame #0 {
      }
      frame #1 {
      }
    }
    n134 = flat-sequence {
      frame #0 {
      }
      frame #1 {
      }
    }
    n135 = property on="Y Position mm PV" class="DigNum (strict)"() -> ("Value"=w286:dbl)  [unwired: 2 in, 2 out]
    n136 = property on="Preset positions" class="Ring (strict)"() -> ("Strings []"=w292:string[])  [unwired: 2 in, 2 out]
    n137 = property on="Z Position mm PV" class="DigNum (strict)"() -> ("Value"=w287:dbl)  [unwired: 2 in, 2 out]
    n138 = property on="X Position mm PV" class="DigNum (strict)"() -> ("Value"=w288:dbl)  [unwired: 2 in, 2 out]
    n139 = event shown="[0] Timeout" {
      selector: _ -> [_ _ _ _ _ _ _ _ _ _ _ _ _ _ _ _ _ _ _ _ _]
      dyn-events: _ -> [_ _ _ _ _ _ _ _ _ _ _ _ _ _ _ _ _ _ _ _ _]
      timeout: 200 -> [_ _ _ _ _ _ _ _ _ _ _ _ _ _ _ _ _ _ _ _ _]
      tunnel: w309 -> [w403 _ _ _ _ _ _ _ _ _ w950 _ _ _ w1180 _ w1247 w1259 w1292 w1358 w1468]
      tunnel: [w402 _ _ _ _ _ _ _ _ _ w956 _ _ _ w1178 _ w1247 w1257 w1294 w1354 w1466] -> w310
      tunnel: w306 -> [w360 _ _ _ _ _ _ _ _ _ w951 _ _ _ w1179 _ w1248 w1260 w1293 w1359 w1469]
      tunnel: [w401 _ _ _ _ _ _ _ _ _ w957 _ _ _ w1175 _ w1248 w1258 w1295 w1355 w1467] -> w308
      tunnel: w305 -> [w359 _ _ _ _ _ _ _ _ _ _ _ w1081 w1141 _ _ _ w1254 w1285 w1361 w1465]
      tunnel: w304 -> [w378 _ _ _ _ _ _ _ _ _ _ _ w1080 w1140 _ _ _ w1253 w1284 w1360 w1464]
      tunnel: [w377 _ _ _ _ _ _ _ _ _ _ _ w1079 w1139 _ _ _ w1256 w1283 w1351 w1463] -> w303
      tunnel: [w376 _ _ _ _ _ _ _ _ _ _ _ w1078 w1138 _ _ _ w1255 w1282 w1350 w1462] -> w302
      tunnel: w301 -> [w361 _ _ _ _ _ _ _ _ _ _ w1013 _ _ _ w1213 _ w1252 w1279 w1357 w1461]
      tunnel: w300 -> [w364 _ _ _ _ _ _ _ _ _ _ w1012 _ _ _ w1212 _ w1251 w1278 w1356 w1460]
      tunnel: [w363 _ _ _ _ _ _ _ _ _ _ w1010 _ _ _ w1210 _ w1250 w1277 w1353 _] -> w299
      tunnel: [w362 _ _ _ _ _ _ _ _ _ _ w1011 _ _ _ w1211 _ w1249 w1276 w1352 _] -> w298
      tunnel: [_ _ _ _ _ _ _ _ _ _ _ _ _ _ _ _ _ _ _ _ w1459] -> w297
      tunnel: [_ _ _ _ _ _ _ _ _ _ _ _ _ _ _ _ _ _ _ _ w1458] -> w296
      event Timeout {
        n140 = event-data() -> ()  [unwired: 1 in, 2 out]
        n141 = property on="X Step SP" class="DigNum (strict)"() -> ("Maximum"=w343:dbl)  [unwired: 2 in, 2 out]
        n142 = property on="Y Step SP" class="DigNum (strict)"() -> ("Maximum"=w348:dbl)  [unwired: 2 in, 2 out]
        n143 = property on="X Step SP" class="DigNum (strict)"() -> ("Minimum"=w344:dbl)  [unwired: 2 in, 2 out]
        n144 = property on="Y Step SP" class="DigNum (strict)"() -> ("Minimum"=w347:dbl)  [unwired: 2 in, 2 out]
        n145 = flat-sequence {
          tunnel: [w413] -> w375
          tunnel: [w426] -> w374
          tunnel: [w435] -> w373
          tunnel: [w406] -> w372
          tunnel: w361 -> [w421]
          tunnel: w364 -> [w422]
          tunnel: w375 -> [w445]
          tunnel: [w445] -> w371
          tunnel: w374 -> [w444]
          tunnel: [w444] -> w370
          tunnel: w373 -> [w443]
          tunnel: [w443] -> w369
          tunnel: w372 -> [w440]
          tunnel: [w440] -> w368
          tunnel: w371 -> [w452]
          tunnel: [w453] -> w367
          tunnel: w370 -> [w455]
          tunnel: [w454] -> w366
          tunnel: w369 -> [w451]
          tunnel: [w450] -> w365
          tunnel: w368 -> [w450]
          tunnel: w367 -> [w465]
          tunnel: w366 -> [w466]
          tunnel: w365 -> [w468]
          tunnel: [w464] -> w362
          tunnel: [w463] -> w363
          frame #0 {
            w425 = 0.2 ("Delay Time (s)")
            n146 = property on="Z Step SP" class="DigNum (strict)"() -> ("Maximum"=w437:dbl)  [unwired: 2 in, 2 out]
            n147 = property on="Z Step SP" class="DigNum (strict)"() -> ("Minimum"=w439:dbl)  [unwired: 2 in, 2 out]
            n148 = property on="Z steps/rev" class="DigNum (strict)"() -> ("Value"=w433:u32)  [unwired: 2 in, 2 out]
            n149 = property on="Z offset mm" class="DigNum (strict)"() -> ("Value"=w429:dbl)  [unwired: 2 in, 2 out]
            n150 = To Long Integer(number=w437) -> (32bit integer=w436:i32)
            n151 = To Long Integer(number=w439) -> (32bit integer=w438:i32)
            n152 = To Double Precision Float(number=w433) -> (double precision float=w434:dbl)
            n153 = call "Applied Send Command.vi"("error in (no error)"=w422, "Command"=T1."Immediate Position?", "VISA resource name"=w421) -> ("error out"=w420:errorcluster, "read buffer"=w417:string, "VISA resource name out"=w415:refnum<visa-resource-name>)  [unwired: 4 in]
            n154 = call "Time Delay17"("error in (no error)"=w420, "Delay Time (s)"=w425) -> ("error out"=w405:errorcluster)  [unwired: 9 in]
            n155 = Hexadecimal String To Number(string=w417, offset=3) -> (number=w418:u32)  [unwired: 1 in, 1 out]
            n156 = To Long Integer(number=w418) -> (32bit integer=w427:i32)
            n157 = call "Applied Send Command.vi"("error in (no error)"=w405, "Command"=T1."Request Status", "VISA resource name"=w415) -> ("error out"=w414:errorcluster, "read buffer"=w410:string, "VISA resource name out"=w413:refnum<visa-resource-name>)  [unwired: 4 in]
            n158 = property on="Z Step PV" class="DigNum (strict)"("Val(Sgnl)"=w427) -> ()  [unwired: 2 in, 2 out]
            n159 = call "Time Delay16"("error in (no error)"=w414, "Delay Time (s)"=w425) -> ("error out"=w426:errorcluster)  [unwired: 9 in]
            n160 = String Subset(string=w410, offset (0)=0, length (rest)=1 ("length (rest)")) -> (substring=w407:string)
            n161 = In Range and Coerce(upper limit=w436, x=w427, lower limit=w438) -> (In Range?=w435:bool)  [unwired: 1 out]
            n162 = To Double Precision Float(number=w427) -> (double precision float=w428:dbl)
            n163 = Not Equal?(x=w407, y="R") -> (x != y?=w406:bool)
            n164 = Equal?(x=w407, y="R") -> (x = y?=w424:bool)
            n165 = property on="Z in Motion" class="Bool (strict)"("Val(Sgnl)"=w406) -> ()  [unwired: 2 in, 2 out]
            n166 = property on="Z in Range" class="Bool (strict)"("Val(Sgnl)"=w435) -> ()  [unwired: 2 in, 2 out]
            n167 = property on="Z Ready" class="Bool (strict)"("Val(Sgnl)"=w424) -> ()  [unwired: 2 in, 2 out]
            n168 = Divide(x=w428, y=w434) -> (x/y=w432:dbl)
            n169 = property on="Z mm/rev" class="DigNum (strict)"() -> ("Value"=w431:dbl)  [unwired: 2 in, 2 out]
            n170 = Multiply(x=w432, y=w431) -> (x*y=w430:dbl)
            n171 = Add(x=w430, y=w429) -> (x+y=w404:dbl)
            n172 = property on="Z Position mm PV" class="DigNum (strict)"("Val(Sgnl)"=w404) -> ()  [unwired: 2 in, 2 out]
            n173 = shared-variable "My Computer\\S132PC1_PV.lvlib\\RZ"(w404) -> ()  [unwired: 1 in, 1 out]
          }
          frame #1 {
            n174 = property on="Z Scan" class="Bool (strict)"() -> ("Value"=w441:bool)  [unwired: 2 in, 2 out]
            n175 = Or(x=w440, y=w441) -> (x .or. y?=w442:bool)
            n176 = case shown="True" w442 {
              frame False {
                n177 = property on="Z Scan OK" class="Bool"("DisabledEnum"=T2."Enabled" ("Disabled")) -> ()  [unwired: 2 in, 2 out]
                n178 = property on="Z Go" class="Bool"("DisabledEnum"=T2."Enabled" ("Disabled")) -> ()  [unwired: 2 in, 2 out]
              }
              frame True {
                n179 = property on="Z Scan OK" class="Bool"("DisabledEnum"=T2."Disabled and Grayed Out" ("Disabled")) -> ()  [unwired: 2 in, 2 out]
                n180 = property on="Z Go" class="Bool"("DisabledEnum"=T2."Disabled and Grayed Out" ("Disabled")) -> ()  [unwired: 2 in, 2 out]
              }
            }
          }
          frame #2 {
            n181 = case shown="False" w451 {
              tunnel: w452 -> [w459 w462]
              tunnel: [w457 w462] -> w453
              tunnel: [w456 w461] -> w454
              tunnel: w455 -> [w458 w461]
              frame False {
                n182 = call "Applied Send Command.vi"("error in (no error)"=w458, "Command"=T1."Stop & Kill Buffer", "VISA resource name"=w459) -> ("error out"=w456:errorcluster, "VISA resource name out"=w457:refnum<visa-resource-name>)  [unwired: 4 in, 1 out]
              }
              frame True {
              }
            }
          }
          frame #3 {
            n183 = property on="Z Backlash corr" class="Bool (strict)"() -> ("Value"=w469:bool)  [unwired: 2 in, 2 out]
            n184 = Implies(1:w468, 2:w469) -> (0:w467:bool)
            n185 = case shown="False" w467 {
              tunnel: w466 -> [w470 w502]
              tunnel: w465 -> [w471 w503]
              tunnel: [w472 w502] -> w464
              tunnel: [w473 w503] -> w463
              frame False {
                w499 = 0.1 ("Delay Time (s)")
                # "Backlash"
                # "Backlash"
                n186 = property on="Z Backlash" class="DigNum (strict)"() -> ("Value"=w477:i32)  [unwired: 2 in, 2 out]
                n187 = property on="Z Backlash corr" class="Bool (strict)"("Val(Sgnl)"=FALSE ("Value (Signaling)")) -> ()  [unwired: 2 in, 2 out]
                n188 = To Long Integer(number=w477) -> (32bit integer=w480:i32)
                n189 = Number To Decimal String(number=w477) -> (decimal integer string=w485:string)  [unwired: 1 in]
                n190 = Negate(x=w480) -> (-x=w479:i32)
                n191 = property on="Z Backlash steps/sec" class="DigNum (strict)"() -> ("Value"=w476:i32)  [unwired: 2 in, 2 out]
                n192 = Number To Decimal String(number=w479) -> (decimal integer string=w486:string)  [unwired: 1 in]
                n193 = property on="Z steps/rev" class="DigNum (strict)"() -> ("Value"=w475:u32)  [unwired: 2 in, 2 out]
                n194 = Divide(x=w476, y=w475) -> (x/y=w500:dbl)
                n195 = Number To Fractional String(number=w500) -> (F-format string=w501:string)  [unwired: 3 in]
                n196 = call "Applied Send Command.vi"("error in (no error)"=w470, "Extra"=w501, "Command"=T1."Velocity Setting", "VISA resource name"=w471) -> ("error out"=w497:errorcluster, "VISA resource name out"=w490:refnum<visa-resource-name>)  [unwired: 3 in, 1 out]
                n197 = call "Time Delay47"("error in (no error)"=w497, "Delay Time (s)"=w499) -> ("error out"=w498:errorcluster)  [unwired: 9 in]
                n198 = call "Applied Send Command.vi"("error in (no error)"=w498, "Extra"=w485, "Command"=T1."Distance or Position", "VISA resource name"=w490) -> ("error out"=w491:errorcluster, "VISA resource name out"=w484:refnum<visa-resource-name>)  [unwired: 3 in, 1 out]
                n199 = call "Time Delay44"("error in (no error)"=w491, "Delay Time (s)"=w499) -> ("error out"=w492:errorcluster)  [unwired: 9 in]
                n200 = call "Applied Send Command.vi"("error in (no error)"=w492, "Command"=T1."Feed to Length", "VISA resource name"=w484) -> ("error out"=w493:errorcluster, "VISA resource name out"=w487:refnum<visa-resource-name>)  [unwired: 4 in, 1 out]
                n201 = call "Time Delay45"("error in (no error)"=w493, "Delay Time (s)"=w499) -> ("error out"=w494:errorcluster)  [unwired: 9 in]
                n202 = call "Applied Send Command.vi"("error in (no error)"=w494, "Extra"=w486, "Command"=T1."Distance or Position", "VISA resource name"=w487) -> ("error out"=w495:errorcluster, "VISA resource name out"=w488:refnum<visa-resource-name>)  [unwired: 3 in, 1 out]
                n203 = call "Time Delay46"("error in (no error)"=w495, "Delay Time (s)"=w499) -> ("error out"=w496:errorcluster)  [unwired: 9 in]
                n204 = call "Applied Send Command.vi"("error in (no error)"=w496, "Command"=T1."Feed to Length", "VISA resource name"=w488) -> ("error out"=w472:errorcluster, "VISA resource name out"=w473:refnum<visa-resource-name>)  [unwired: 4 in, 1 out]
              }
              frame True {
              }
            }
          }
        }
        n205 = property on="X Step PV" class="DigNum (strict)"() -> ("Value"=w342:i32)  [unwired: 2 in, 2 out]
        n206 = property on="Y Step PV" class="DigNum (strict)"() -> ("Value"=w341:i32)  [unwired: 2 in, 2 out]
        n207 = Subtract(x=w343, y=w344) -> (x-y=w345:dbl)
        n208 = Absolute Value(x=w342) -> (abs(x)=w339:i32)
        n209 = Absolute Value(x=w341) -> (abs(x)=w340:i32)
        n210 = Subtract(x=w348, y=w347) -> (x-y=w349:dbl)
        n211 = property on="Y Scan Length SP steps" class="DigNum (strict)"() -> ("Value"=w351:i32)  [unwired: 2 in, 2 out]
        n212 = property on="Z Scan Length SP steps" class="DigNum (strict)"() -> ("Value"=w352:i32)  [unwired: 2 in, 2 out]
        n213 = Multiply(x=w339, y=w340) -> (x*y=w334:i32)
        n214 = Divide(x=w349, y=2.0) -> (x/y=w337:dbl)
        n215 = Divide(x=w345, y=2.0) -> (x/y=w338:dbl)
        n216 = Absolute Value(x=w337) -> (abs(x)=w335:dbl)
        n217 = Absolute Value(x=w338) -> (abs(x)=w336:dbl)
        n218 = Divide(x=w351, y=w352) -> (x/y=w353:dbl)
        n219 = Multiply(x=w335, y=w336) -> (x*y=w333:dbl)
        n220 = Inverse Tangent(1:w353) -> (0:w354:dbl)
        n221 = Less Or Equal?(x=w334, y=w333) -> (x <= y?=w332:bool)
        n222 = Divide(x=w354, y=6.283185307179586) -> (x/y=w355:dbl)
        n223 = flat-sequence {
          tunnel: [w517] -> w389
          tunnel: [w528] -> w388
          tunnel: [w506] -> w387
          tunnel: [w513] -> w386
          tunnel: w359 -> [w524]
          tunnel: w378 -> [w512]
          tunnel: w343 -> [w508]
          tunnel: w344 -> [w507]
          tunnel: w332 -> [w505]
          tunnel: w389 -> [w547]
          tunnel: [w547] -> w385
          tunnel: w388 -> [w546]
          tunnel: [w546] -> w384
          tunnel: w387 -> [w545]
          tunnel: [w545] -> w383
          tunnel: w386 -> [w542]
          tunnel: [w542] -> w382
          tunnel: w385 -> [w556]
          tunnel: [w553] -> w381
          tunnel: w384 -> [w555]
          tunnel: [w554] -> w380
          tunnel: w383 -> [w552]
          tunnel: [w557] -> w379
          tunnel: w382 -> [w557]
          tunnel: w381 -> [w568]
          tunnel: w380 -> [w569]
          tunnel: w379 -> [w570]
          tunnel: [w567] -> w376
          tunnel: [w566] -> w377
          frame #0 {
            w527 = 0.2 ("Delay Time (s)")
            n224 = To Long Integer(number=w508) -> (32bit integer=w539:i32)
            n225 = To Long Integer(number=w507) -> (32bit integer=w540:i32)
            n226 = property on="X steps/rev" class="DigNum (strict)"() -> ("Value"=w536:u32)  [unwired: 2 in, 2 out]
            n227 = property on="X offset mm" class="DigNum (strict)"() -> ("Value"=w532:dbl)  [unwired: 2 in, 2 out]
            n228 = To Double Precision Float(number=w536) -> (double precision float=w537:dbl)
            n229 = call "Applied Send Command.vi"("error in (no error)"=w512, "Command"=T1."Immediate Position?", "VISA resource name"=w524) -> ("error out"=w522:errorcluster, "read buffer"=w523:string, "VISA resource name out"=w518:refnum<visa-resource-name>)  [unwired: 4 in]
            n230 = call "Time Delay12"("error in (no error)"=w522, "Delay Time (s)"=w527) -> ("error out"=w515:errorcluster)  [unwired: 9 in]
            n231 = Hexadecimal String To Number(string=w523, offset=3) -> (number=w529:u32)  [unwired: 1 in, 1 out]
            n232 = To Long Integer(number=w529) -> (32bit integer=w530:i32)
            n233 = call "Applied Send Command.vi"("error in (no error)"=w515, "Command"=T1."Request Status", "VISA resource name"=w518) -> ("error out"=w516:errorcluster, "read buffer"=w520:string, "VISA resource name out"=w517:refnum<visa-resource-name>)  [unwired: 4 in]
            n234 = property on="X Step PV" class="DigNum (strict)"("Val(Sgnl)"=w530) -> ()  [unwired: 2 in, 2 out]
            n235 = call "Time Delay11"("error in (no error)"=w516, "Delay Time (s)"=w527) -> ("error out"=w528:errorcluster)  [unwired: 9 in]
            n236 = String Subset(string=w520, offset (0)=0, length (rest)=1 ("length (rest)")) -> (substring=w509:string)
            n237 = In Range and Coerce(upper limit=w539, x=w530, lower limit=w540) -> (In Range?=w538:bool)  [unwired: 1 out]
            n238 = To Double Precision Float(number=w530) -> (double precision float=w531:dbl)
            n239 = Not Equal?(x=w509, y="R") -> (x != y?=w513:bool)
            n240 = Equal?(x=w509, y="R") -> (x = y?=w526:bool)
            n241 = property on="X  in Motion" class="Bool (strict)"("Val(Sgnl)"=w513) -> ()  [unwired: 2 in, 2 out]
            n242 = property on="X Ready" class="Bool (strict)"("Val(Sgnl)"=w526) -> ()  [unwired: 2 in, 2 out]
            n243 = Divide(x=w531, y=w537) -> (x/y=w535:dbl)
            n244 = And(x=w505, y=w538) -> (x .and. y?=w506:bool)
            n245 = property on="X  in Range" class="Bool (strict)"("Val(Sgnl)"=w506) -> ()  [unwired: 2 in, 2 out]
            n246 = property on="X mm/rev" class="DigNum (strict)"() -> ("Value"=w534:dbl)  [unwired: 2 in, 2 out]
            n247 = Multiply(x=w535, y=w534) -> (x*y=w533:dbl)
            n248 = Add(x=w533, y=w532) -> (x+y=w504:dbl)
            n249 = shared-variable "My Computer\\S132PC1_PV.lvlib\\RX"(w504) -> ()  [unwired: 1 in, 1 out]
            n250 = property on="X Position mm PV" class="DigNum (strict)"("Val(Sgnl)"=w504) -> ()  [unwired: 2 in, 2 out]
          }
          frame #1 {
            n251 = property on="X Scan" class="Bool (strict)"() -> ("Value"=w543:bool)  [unwired: 2 in, 2 out]
            n252 = Or(x=w542, y=w543) -> (x .or. y?=w544:bool)
            n253 = case shown="True" w544 {
              frame False {
                n254 = property on="X Scan OK" class="Bool"("DisabledEnum"=T2."Enabled" ("Disabled")) -> ()  [unwired: 2 in, 2 out]
                n255 = property on="X Go" class="Bool"("DisabledEnum"=T2."Enabled" ("Disabled")) -> ()  [unwired: 2 in, 2 out]
              }
              frame True {
                n256 = property on="X Scan OK" class="Bool"("DisabledEnum"=T2."Disabled and Grayed Out" ("Disabled")) -> ()  [unwired: 2 in, 2 out]
                n257 = property on="X Go" class="Bool"("DisabledEnum"=T2."Disabled and Grayed Out" ("Disabled")) -> ()  [unwired: 2 in, 2 out]
              }
            }
          }
          frame #2 {
            n258 = case shown="False" w552 {
              tunnel: w556 -> [w559 w564]
              tunnel: [w561 w564] -> w553
              tunnel: [w562 w563] -> w554
              tunnel: w555 -> [w558 w563]
              frame False {
                n259 = call "Applied Send Command.vi"("error in (no error)"=w558, "Command"=T1."Stop & Kill Buffer", "VISA resource name"=w559) -> ("error out"=w562:errorcluster, "VISA resource name out"=w561:refnum<visa-resource-name>)  [unwired: 4 in, 1 out]
              }
              frame True {
              }
            }
          }
          frame #3 {
            n260 = property on="X Backlash corr" class="Bool (strict)"() -> ("Value"=w571:bool)  [unwired: 2 in, 2 out]
            n261 = Implies(1:w570, 2:w571) -> (0:w565:bool)
            n262 = case shown="False" w565 {
              tunnel: w569 -> [w585 w604]
              tunnel: w568 -> [w586 w605]
              tunnel: [w588 w604] -> w567
              tunnel: [w587 w605] -> w566
              frame False {
                w576 = 0.1 ("Delay Time (s)")
                # "Backlash"
                n263 = property on="X Backlash" class="DigNum (strict)"() -> ("Value"=w591:i32)  [unwired: 2 in, 2 out]
                n264 = property on="X Backlash corr" class="Bool (strict)"("Val(Sgnl)"=FALSE ("Value (Signaling)")) -> ()  [unwired: 2 in, 2 out]
                n265 = To Long Integer(number=w591) -> (32bit integer=w600:i32)
                n266 = Number To Decimal String(number=w591) -> (decimal integer string=w595:string)  [unwired: 1 in]
                n267 = Negate(x=w600) -> (-x=w601:i32)
                n268 = property on="X Backlash steps/sec" class="DigNum (strict)"() -> ("Value"=w575:i32)  [unwired: 2 in, 2 out]
                n269 = Number To Decimal String(number=w601) -> (decimal integer string=w594:string)  [unwired: 1 in]
                n270 = property on="X steps/rev" class="DigNum (strict)"() -> ("Value"=w574:u32)  [unwired: 2 in, 2 out]
                n271 = Divide(x=w575, y=w574) -> (x/y=w573:dbl)
                n272 = Number To Fractional String(number=w573) -> (F-format string=w572:string)  [unwired: 3 in]
                n273 = call "Applied Send Command.vi"("error in (no error)"=w585, "Extra"=w572, "Command"=T1."Velocity Setting", "VISA resource name"=w586) -> ("error out"=w578:errorcluster, "VISA resource name out"=w589:refnum<visa-resource-name>)  [unwired: 3 in, 1 out]
                n274 = call "Time Delay35"("error in (no error)"=w578, "Delay Time (s)"=w576) -> ("error out"=w577:errorcluster)  [unwired: 9 in]
                n275 = call "Applied Send Command.vi"("error in (no error)"=w577, "Extra"=w595, "Command"=T1."Distance or Position", "VISA resource name"=w589) -> ("error out"=w584:errorcluster, "VISA resource name out"=w596:refnum<visa-resource-name>)  [unwired: 3 in, 1 out]
                n276 = call "Time Delay32"("error in (no error)"=w584, "Delay Time (s)"=w576) -> ("error out"=w583:errorcluster)  [unwired: 9 in]
                n277 = call "Applied Send Command.vi"("error in (no error)"=w583, "Command"=T1."Feed to Length", "VISA resource name"=w596) -> ("error out"=w582:errorcluster, "VISA resource name out"=w593:refnum<visa-resource-name>)  [unwired: 4 in, 1 out]
                n278 = call "Time Delay33"("error in (no error)"=w582, "Delay Time (s)"=w576) -> ("error out"=w581:errorcluster)  [unwired: 9 in]
                n279 = call "Applied Send Command.vi"("error in (no error)"=w581, "Extra"=w594, "Command"=T1."Distance or Position", "VISA resource name"=w593) -> ("error out"=w580:errorcluster, "VISA resource name out"=w592:refnum<visa-resource-name>)  [unwired: 3 in, 1 out]
                n280 = call "Time Delay34"("error in (no error)"=w580, "Delay Time (s)"=w576) -> ("error out"=w579:errorcluster)  [unwired: 9 in]
                n281 = call "Applied Send Command.vi"("error in (no error)"=w579, "Command"=T1."Feed to Length", "VISA resource name"=w592) -> ("error out"=w588:errorcluster, "VISA resource name out"=w587:refnum<visa-resource-name>)  [unwired: 4 in, 1 out]
              }
              frame True {
              }
            }
          }
        }
        n282 = flat-sequence {
          tunnel: w403 -> [w623]
          tunnel: w360 -> [w624]
          tunnel: [w620] -> w400
          tunnel: [w630] -> w398
          tunnel: [w609] -> w396
          tunnel: [w611] -> w394
          tunnel: w348 -> [w610]
          tunnel: w347 -> [w607]
          tunnel: w332 -> [w608]
          tunnel: w400 -> [w649]
          tunnel: [w649] -> w399
          tunnel: w398 -> [w648]
          tunnel: [w648] -> w397
          tunnel: w396 -> [w647]
          tunnel: [w647] -> w395
          tunnel: w394 -> [w644]
          tunnel: [w644] -> w390
          tunnel: w399 -> [w656]
          tunnel: [w657] -> w393
          tunnel: w397 -> [w659]
          tunnel: [w658] -> w392
          tunnel: w395 -> [w655]
          tunnel: [w654] -> w391
          tunnel: w390 -> [w654]
          tunnel: w393 -> [w669]
          tunnel: w392 -> [w670]
          tunnel: w391 -> [w672]
          tunnel: [w668] -> w402
          tunnel: [w667] -> w401
          frame #0 {
            w629 = 0.2 ("Delay Time (s)")
            n283 = To Long Integer(number=w610) -> (32bit integer=w641:i32)
            n284 = To Long Integer(number=w607) -> (32bit integer=w642:i32)
            n285 = property on="Y steps/rev" class="DigNum (strict)"() -> ("Value"=w638:u32)  [unwired: 2 in, 2 out]
            n286 = property on="Y offset mm" class="DigNum (strict)"() -> ("Value"=w634:dbl)  [unwired: 2 in, 2 out]
            n287 = To Double Precision Float(number=w638) -> (double precision float=w639:dbl)
            n288 = call "Applied Send Command.vi"("error in (no error)"=w623, "Command"=T1."Immediate Position?", "VISA resource name"=w624) -> ("error out"=w626:errorcluster, "read buffer"=w627:string, "VISA resource name out"=w621:refnum<visa-resource-name>)  [unwired: 4 in]
            n289 = call "Time Delay4"("error in (no error)"=w626, "Delay Time (s)"=w629) -> ("error out"=w619:errorcluster)  [unwired: 9 in]
            n290 = Hexadecimal String To Number(string=w627, offset=3) -> (number=w631:u32)  [unwired: 1 in, 1 out]
            n291 = To Long Integer(number=w631) -> (32bit integer=w632:i32)
            n292 = call "Applied Send Command.vi"("error in (no error)"=w619, "Command"=T1."Request Status", "VISA resource name"=w621) -> ("error out"=w618:errorcluster, "read buffer"=w615:string, "VISA resource name out"=w620:refnum<visa-resource-name>)  [unwired: 4 in]
            n293 = property on="Y Step PV" class="DigNum (strict)"("Val(Sgnl)"=w632) -> ()  [unwired: 2 in, 2 out]
            n294 = call "Time Delay3"("error in (no error)"=w618, "Delay Time (s)"=w629) -> ("error out"=w630:errorcluster)  [unwired: 9 in]
            n295 = String Subset(string=w615, offset (0)=0, length (rest)=1 ("length (rest)")) -> (substring=w613:string)
            n296 = In Range and Coerce(upper limit=w641, x=w632, lower limit=w642) -> (In Range?=w640:bool)  [unwired: 1 out]
            n297 = To Double Precision Float(number=w632) -> (double precision float=w633:dbl)
            n298 = Not Equal?(x=w613, y="R") -> (x != y?=w611:bool)
            n299 = Equal?(x=w613, y="R") -> (x = y?=w628:bool)
            n300 = property on="Y in Motion" class="Bool (strict)"("Val(Sgnl)"=w611) -> ()  [unwired: 2 in, 2 out]
            n301 = property on="Y Ready" class="Bool (strict)"("Val(Sgnl)"=w628) -> ()  [unwired: 2 in, 2 out]
            n302 = Divide(x=w633, y=w639) -> (x/y=w637:dbl)
            n303 = And(x=w640, y=w608) -> (x .and. y?=w609:bool)
            n304 = property on="Y in Range" class="Bool (strict)"("Val(Sgnl)"=w609) -> ()  [unwired: 2 in, 2 out]
            n305 = property on="Y mm/rev" class="DigNum (strict)"() -> ("Value"=w636:dbl)  [unwired: 2 in, 2 out]
            n306 = Multiply(x=w637, y=w636) -> (x*y=w635:dbl)
            n307 = Add(x=w635, y=w634) -> (x+y=w606:dbl)
            n308 = property on="Y Position mm PV" class="DigNum (strict)"("Val(Sgnl)"=w606) -> ()  [unwired: 2 in, 2 out]
            n309 = shared-variable "My Computer\\S132PC1_PV.lvlib\\RY"(w606) -> ()  [unwired: 1 in, 1 out]
          }
          frame #1 {
            n310 = property on="Y Scan" class="Bool (strict)"() -> ("Value"=w645:bool)  [unwired: 2 in, 2 out]
            n311 = Or(x=w644, y=w645) -> (x .or. y?=w646:bool)
            n312 = case shown="True" w646 {
              frame False {
                n313 = property on="Y Scan OK" class="Bool"("DisabledEnum"=T2."Enabled" ("Disabled")) -> ()  [unwired: 2 in, 2 out]
                n314 = property on="Y Go" class="Bool"("DisabledEnum"=T2."Enabled" ("Disabled")) -> ()  [unwired: 2 in, 2 out]
              }
              frame True {
                n315 = property on="Y Scan OK" class="Bool"("DisabledEnum"=T2."Disabled and Grayed Out" ("Disabled")) -> ()  [unwired: 2 in, 2 out]
                n316 = property on="Y Go" class="Bool"("DisabledEnum"=T2."Disabled and Grayed Out" ("Disabled")) -> ()  [unwired: 2 in, 2 out]
              }
            }
          }
          frame #2 {
            n317 = case shown="False" w655 {
              tunnel: w656 -> [w661 w666]
              tunnel: [w663 w666] -> w657
              tunnel: [w662 w665] -> w658
              tunnel: w659 -> [w660 w665]
              frame False {
                n318 = call "Applied Send Command.vi"("error in (no error)"=w660, "Command"=T1."Stop & Kill Buffer", "VISA resource name"=w661) -> ("error out"=w662:errorcluster, "VISA resource name out"=w663:refnum<visa-resource-name>)  [unwired: 4 in, 1 out]
              }
              frame True {
              }
            }
          }
          frame #3 {
            n319 = property on="Y Backlash corr" class="Bool (strict)"() -> ("Value"=w673:bool)  [unwired: 2 in, 2 out]
            n320 = Implies(1:w672, 2:w673) -> (0:w671:bool)
            n321 = case shown="False" w671 {
              tunnel: w670 -> [w676 w705]
              tunnel: w669 -> [w677 w706]
              tunnel: [w674 w705] -> w668
              tunnel: [w675 w706] -> w667
              frame False {
                w683 = 0.1 ("Delay Time (s)")
                # "Backlash"
                n322 = property on="Y Backlash" class="DigNum (strict)"() -> ("Value"=w678:i32)  [unwired: 2 in, 2 out]
                n323 = property on="Y Backlash corr" class="Bool (strict)"("Val(Sgnl)"=FALSE ("Value (Signaling)")) -> ()  [unwired: 2 in, 2 out]
                n324 = To Long Integer(number=w678) -> (32bit integer=w701:i32)
                n325 = Number To Decimal String(number=w678) -> (decimal integer string=w696:string)  [unwired: 1 in]
                n326 = Negate(x=w701) -> (-x=w702:i32)
                n327 = property on="Y Backlash steps/sec" class="DigNum (strict)"() -> ("Value"=w679:i32)  [unwired: 2 in, 2 out]
                n328 = Number To Decimal String(number=w702) -> (decimal integer string=w695:string)  [unwired: 1 in]
                n329 = property on="Y steps/rev" class="DigNum (strict)"() -> ("Value"=w682:u32)  [unwired: 2 in, 2 out]
                n330 = Divide(x=w679, y=w682) -> (x/y=w681:dbl)
                n331 = Number To Fractional String(number=w681) -> (F-format string=w680:string)  [unwired: 3 in]
                n332 = call "Applied Send Command.vi"("error in (no error)"=w676, "Extra"=w680, "Command"=T1."Velocity Setting", "VISA resource name"=w677) -> ("error out"=w685:errorcluster, "VISA resource name out"=w691:refnum<visa-resource-name>)  [unwired: 3 in, 1 out]
                n333 = call "Time Delay41"("error in (no error)"=w685, "Delay Time (s)"=w683) -> ("error out"=w684:errorcluster)  [unwired: 9 in]
                n334 = call "Applied Send Command.vi"("error in (no error)"=w684, "Extra"=w696, "Command"=T1."Distance or Position", "VISA resource name"=w691) -> ("error out"=w690:errorcluster, "VISA resource name out"=w697:refnum<visa-resource-name>)  [unwired: 3 in, 1 out]
                n335 = call "Time Delay38"("error in (no error)"=w690, "Delay Time (s)"=w683) -> ("error out"=w689:errorcluster)  [unwired: 9 in]
                n336 = call "Applied Send Command.vi"("error in (no error)"=w689, "Command"=T1."Feed to Length", "VISA resource name"=w697) -> ("error out"=w688:errorcluster, "VISA resource name out"=w694:refnum<visa-resource-name>)  [unwired: 4 in, 1 out]
                n337 = call "Applied Send Command.vi"("Extra"=w695, "Command"=T1."Distance or Position", "VISA resource name"=w694) -> ("error out"=w687:errorcluster, "VISA resource name out"=w693:refnum<visa-resource-name>)  [unwired: 4 in, 1 out]
                n338 = call "Time Delay39"("error in (no error)"=w688, "Delay Time (s)"=w683) -> ()  [unwired: 9 in, 1 out]
                n339 = call "Time Delay40"("error in (no error)"=w687, "Delay Time (s)"=w683) -> ("error out"=w686:errorcluster)  [unwired: 9 in]
                n340 = call "Applied Send Command.vi"("error in (no error)"=w686, "Command"=T1."Feed to Length", "VISA resource name"=w693) -> ("error out"=w674:errorcluster, "VISA resource name out"=w675:refnum<visa-resource-name>)  [unwired: 4 in, 1 out]
              }
              frame True {
              }
            }
          }
        }
        n341 = Multiply(x=360.0, y=w355) -> (x*y=w358:dbl)
        n342 = property on="atan Y/Z" class="DigNum (strict)"("Val(Sgnl)"=w358) -> ()  [unwired: 2 in, 2 out]
      }
      event "Reset Y Position mm", "Reset X Position mm", "Reset Z Position mm": Value Change {
        n343 = event-data() -> ()  [unwired: 1 in, 5 out]
        n344 = property on="Z steps/rev" class="DigNum (strict)"() -> ("Value"=w709:u32)  [unwired: 2 in, 2 out]
        n345 = property on="X steps/rev" class="DigNum (strict)"() -> ("Value"=w718:u32)  [unwired: 2 in, 2 out]
        n346 = property on="Y steps/rev" class="DigNum (strict)"() -> ("Value"=w727:u32)  [unwired: 2 in, 2 out]
        n347 = property on="Z offset mm" class="DigNum (strict)"() -> ("Value"=w707:dbl)  [unwired: 2 in, 2 out]
        n348 = property on="X offset mm" class="DigNum (strict)"() -> ("Value"=w716:dbl)  [unwired: 2 in, 2 out]
        n349 = property on="Y offset mm" class="DigNum (strict)"() -> ("Value"=w725:dbl)  [unwired: 2 in, 2 out]
        n350 = To Double Precision Float(number=w718) -> (double precision float=w721:dbl)
        n351 = To Double Precision Float(number=w727) -> (double precision float=w730:dbl)
        n352 = property on="Reset Z Position mm" class="DigNum (strict)"() -> ("Value"=w715:dbl)  [unwired: 2 in, 2 out]
        n353 = property on="Reset X Position mm" class="DigNum (strict)"() -> ("Value"=w724:dbl)  [unwired: 2 in, 2 out]
        n354 = property on="Reset Y Position mm" class="DigNum (strict)"() -> ("Value"=w733:dbl)  [unwired: 2 in, 2 out]
        n355 = Subtract(x=w715, y=w707) -> (x-y=w714:dbl)
        n356 = Subtract(x=w724, y=w716) -> (x-y=w723:dbl)
        n357 = Subtract(x=w733, y=w725) -> (x-y=w732:dbl)
        n358 = property on="Z mm/rev" class="DigNum (strict)"() -> ("Value"=w708:dbl)  [unwired: 2 in, 2 out]
        n359 = property on="X mm/rev" class="DigNum (strict)"() -> ("Value"=w717:dbl)  [unwired: 2 in, 2 out]
        n360 = property on="Y mm/rev" class="DigNum (strict)"() -> ("Value"=w726:dbl)  [unwired: 2 in, 2 out]
        n361 = Divide(x=w723, y=w717) -> (x/y=w722:dbl)
        n362 = Divide(x=w732, y=w726) -> (x/y=w731:dbl)
        n363 = Divide(x=w714, y=w708) -> (x/y=w713:dbl)
        n364 = To Double Precision Float(number=w709) -> (double precision float=w712:dbl)
        n365 = Multiply(x=w713, y=w712) -> (x*y=w711:dbl)
        n366 = Multiply(x=w722, y=w721) -> (x*y=w720:dbl)
        n367 = Multiply(x=w731, y=w730) -> (x*y=w729:dbl)
        n368 = To Long Integer(number=w711) -> (32bit integer=w710:i32)
        n369 = To Long Integer(number=w720) -> (32bit integer=w719:i32)
        n370 = To Long Integer(number=w729) -> (32bit integer=w728:i32)
        n371 = property on="Reset Z Motor Steps" class="DigNum (strict)"("Val(Sgnl)"=w710) -> ()  [unwired: 2 in, 2 out]
        n372 = property on="Reset X Motor Steps" class="DigNum (strict)"("Val(Sgnl)"=w719) -> ()  [unwired: 2 in, 2 out]
        n373 = property on="Reset Y Motor Steps" class="DigNum (strict)"("Val(Sgnl)"=w728) -> ()  [unwired: 2 in, 2 out]
      }
      event "Y Velocity SP step/sec", "X Velocity SP step/sec", "Z Velocity SP step/sec", "Y Step SP", "X Step SP", "Z Step SP": Value Change {
        n374 = event-data() -> ()  [unwired: 1 in, 5 out]
        n375 = property on="Z Step SP" class="DigNum (strict)"() -> ("Value"=w740:i32)  [unwired: 2 in, 2 out]
        n376 = property on="Y Step SP" class="DigNum (strict)"() -> ("Value"=w756:i32)  [unwired: 2 in, 2 out]
        n377 = property on="X Step SP" class="DigNum (strict)"() -> ("Value"=w748:i32)  [unwired: 2 in, 2 out]
        n378 = property on="Z steps/rev" class="DigNum (strict)"() -> ("Value"=w761:u32)  [unwired: 2 in, 2 out]
        n379 = property on="Z steps/rev" class="DigNum (strict)"() -> ("Value"=w738:u32)  [unwired: 2 in, 2 out]
        n380 = property on="Y steps/rev" class="DigNum (strict)"() -> ("Value"=w773:u32)  [unwired: 2 in, 2 out]
        n381 = property on="Y steps/rev" class="DigNum (strict)"() -> ("Value"=w754:u32)  [unwired: 2 in, 2 out]
        n382 = property on="X steps/rev" class="DigNum (strict)"() -> ("Value"=w767:u32)  [unwired: 2 in, 2 out]
        n383 = property on="X steps/rev" class="DigNum (strict)"() -> ("Value"=w746:u32)  [unwired: 2 in, 2 out]
        n384 = property on="Z offset mm" class="DigNum (strict)"() -> ("Value"=w737:dbl)  [unwired: 2 in, 2 out]
        n385 = property on="Y offset mm" class="DigNum (strict)"() -> ("Value"=w753:dbl)  [unwired: 2 in, 2 out]
        n386 = property on="X offset mm" class="DigNum (strict)"() -> ("Value"=w745:dbl)  [unwired: 2 in, 2 out]
        n387 = To Double Precision Float(number=w761) -> (double precision float=w766:dbl)
        n388 = To Double Precision Float(number=w740) -> (double precision float=w741:dbl)
        n389 = To Double Precision Float(number=w738) -> (double precision float=w744:dbl)
        n390 = To Double Precision Float(number=w756) -> (double precision float=w757:dbl)
        n391 = To Double Precision Float(number=w754) -> (double precision float=w760:dbl)
        n392 = To Double Precision Float(number=w767) -> (double precision float=w772:dbl)
        n393 = To Double Precision Float(number=w748) -> (double precision float=w749:dbl)
        n394 = To Double Precision Float(number=w746) -> (double precision float=w752:dbl)
        n395 = Divide(x=w741, y=w744) -> (x/y=w743:dbl)
        n396 = Divide(x=w757, y=w760) -> (x/y=w759:dbl)
        n397 = Divide(x=w749, y=w752) -> (x/y=w751:dbl)
        n398 = property on="Z Velocity SP step/sec" class="DigNum (strict)"() -> ("Value"=w763:i32)  [unwired: 2 in, 2 out]
        n399 = property on="Z mm/rev" class="DigNum (strict)"() -> ("Value"=w736:dbl)  [unwired: 2 in, 2 out]
        n400 = property on="Y Velocity SP step/sec" class="DigNum (strict)"() -> ("Value"=w775:i32)  [unwired: 2 in, 2 out]
        n401 = property on="Y mm/rev" class="DigNum (strict)"() -> ("Value"=w734:dbl)  [unwired: 2 in, 2 out]
        n402 = property on="X Velocity SP step/sec" class="DigNum (strict)"() -> ("Value"=w769:i32)  [unwired: 2 in, 2 out]
        n403 = property on="X mm/rev" class="DigNum (strict)"() -> ("Value"=w735:dbl)  [unwired: 2 in, 2 out]
        n404 = Multiply(x=w743, y=w736) -> (x*y=w742:dbl)
        n405 = Multiply(x=w759, y=w734) -> (x*y=w758:dbl)
        n406 = Multiply(x=w751, y=w735) -> (x*y=w750:dbl)
        n407 = To Double Precision Float(number=w763) -> (double precision float=w764:dbl)
        n408 = To Double Precision Float(number=w775) -> (double precision float=w776:dbl)
        n409 = To Double Precision Float(number=w773) -> (double precision float=w778:dbl)
        n410 = To Double Precision Float(number=w769) -> (double precision float=w770:dbl)
        n411 = Divide(x=w764, y=w766) -> (x/y=w765:dbl)
        n412 = Add(x=w742, y=w737) -> (x+y=w739:dbl)
        n413 = Divide(x=w776, y=w778) -> (x/y=w777:dbl)
        n414 = Add(x=w758, y=w753) -> (x+y=w755:dbl)
        n415 = Divide(x=w770, y=w772) -> (x/y=w771:dbl)
        n416 = Add(x=w750, y=w745) -> (x+y=w747:dbl)
        n417 = Multiply(x=w765, y=w736) -> (x*y=w762:dbl)
        n418 = property on="Z Position MV mm" class="DigNum (strict)"("Val(Sgnl)"=w739) -> ()  [unwired: 2 in, 2 out]
        n419 = Multiply(x=w777, y=w734) -> (x*y=w774:dbl)
        n420 = property on="Y Position MV mm" class="DigNum (strict)"("Val(Sgnl)"=w755) -> ()  [unwired: 2 in, 2 out]
        n421 = Multiply(x=w771, y=w735) -> (x*y=w768:dbl)
        n422 = property on="X Position MV mm" class="DigNum (strict)"("Val(Sgnl)"=w747) -> ()  [unwired: 2 in, 2 out]
        n423 = property on="Z Velocity MV mm/sec" class="DigNum (strict)"("Val(Sgnl)"=w762) -> ()  [unwired: 2 in, 2 out]
        n424 = property on="Y Velocity MV mm/sec" class="DigNum (strict)"("Val(Sgnl)"=w774) -> ()  [unwired: 2 in, 2 out]
        n425 = property on="X Velocity MV mm/sec" class="DigNum (strict)"("Val(Sgnl)"=w768) -> ()  [unwired: 2 in, 2 out]
      }
      event "Y Scan Length SP steps", "Y Scan Velocity SP steps/sec", "X Scan Velocity SP steps/sec", "X Scan Length SP steps", "Z Scan Velocity SP steps/sec", "Z Scan Length SP steps": Value Change {
        n426 = event-data() -> ()  [unwired: 1 in, 5 out]
        n427 = property on="Z steps/rev" class="DigNum (strict)"() -> ("Value"=w802:u32)  [unwired: 2 in, 2 out]
        n428 = property on="X steps/rev" class="DigNum (strict)"() -> ("Value"=w829:u32)  [unwired: 2 in, 2 out]
        n429 = property on="Y steps/rev" class="DigNum (strict)"() -> ("Value"=w815:u32)  [unwired: 2 in, 2 out]
        n430 = property on="X Step PV" class="DigNum (strict)"() -> ("Value"=w827:i32)  [unwired: 2 in, 2 out]
        n431 = property on="Y Step PV" class="DigNum (strict)"() -> ("Value"=w813:i32)  [unwired: 2 in, 2 out]
        n432 = property on="Z Step PV" class="DigNum (strict)"() -> ("Value"=w800:i32)  [unwired: 2 in, 2 out]
        n433 = To Double Precision Float(number=w827) -> (double precision float=w794:dbl)
        n434 = To Double Precision Float(number=w813) -> (double precision float=w793:dbl)
        n435 = To Double Precision Float(number=w800) -> (double precision float=w792:dbl)
        n436 = To Double Precision Float(number=w802) -> (double precision float=w799:dbl)
        n437 = To Double Precision Float(number=w829) -> (double precision float=w826:dbl)
        n438 = To Double Precision Float(number=w815) -> (double precision float=w788:dbl)
        n439 = property on="X Step SP" class="DigNum (strict)"() -> ("Maximum"=w833:dbl)  [unwired: 2 in, 2 out]
        n440 = property on="Y Step SP" class="DigNum (strict)"() -> ("Maximum"=w819:dbl)  [unwired: 2 in, 2 out]
        n441 = property on="Z Step SP" class="DigNum (strict)"() -> ("Maximum"=w806:dbl)  [unwired: 2 in, 2 out]
        n442 = property on="X Step SP" class="DigNum (strict)"() -> ("Minimum"=w834:dbl)  [unwired: 2 in, 2 out]
        n443 = property on="Y Step SP" class="DigNum (strict)"() -> ("Minimum"=w820:dbl)  [unwired: 2 in, 2 out]
        n444 = property on="Z Step SP" class="DigNum (strict)"() -> ("Minimum"=w807:dbl)  [unwired: 2 in, 2 out]
        n445 = property on="Z Scan Length SP steps" class="DigNum (strict)"() -> ("Value"=w803:i32)  [unwired: 2 in, 2 out]
        n446 = property on="X Scan Length SP steps" class="DigNum (strict)"() -> ("Value"=w825:i32)  [unwired: 2 in, 2 out]
        n447 = property on="Y Scan Length SP steps" class="DigNum (strict)"() -> ("Value"=w816:i32)  [unwired: 2 in, 2 out]
        n448 = property on="Z Scan Velocity SP steps/sec" class="DigNum (strict)"() -> ("Value"=w798:i32)  [unwired: 2 in, 2 out]
        n449 = property on="X Scan Velocity SP steps/sec" class="DigNum (strict)"() -> ("Value"=w830:i32)  [unwired: 2 in, 2 out]
        n450 = property on="Y Scan Velocity SP steps/sec" class="DigNum (strict)"() -> ("Value"=w812:i32)  [unwired: 2 in, 2 out]
        n451 = Subtract(x=w834, y=w794) -> (x-y=w835:dbl)
        n452 = Subtract(x=w833, y=w794) -> (x-y=w832:dbl)
        n453 = Subtract(x=w820, y=w793) -> (x-y=w821:dbl)
        n454 = Subtract(x=w819, y=w793) -> (x-y=w818:dbl)
        n455 = Subtract(x=w807, y=w792) -> (x-y=w808:dbl)
        n456 = Subtract(x=w806, y=w792) -> (x-y=w805:dbl)
        n457 = To Double Precision Float(number=w803) -> (double precision float=w791:dbl)
        n458 = To Double Precision Float(number=w825) -> (double precision float=w783:dbl)
        n459 = To Double Precision Float(number=w816) -> (double precision float=w787:dbl)
        n460 = property on="X Scan Length SP steps" class="DigNum (strict)"("Minimum"=w835) -> ()  [unwired: 2 in, 2 out]
        n461 = property on="Y Scan Length SP steps" class="DigNum (strict)"("Minimum"=w821) -> ()  [unwired: 2 in, 2 out]
        n462 = property on="Z Scan Length SP steps" class="DigNum (strict)"("Minimum"=w808) -> ()  [unwired: 2 in, 2 out]
        n463 = property on="X Scan Length SP steps" class="DigNum (strict)"("Maximum"=w832) -> ()  [unwired: 2 in, 2 out]
        n464 = property on="Y Scan Length SP steps" class="DigNum (strict)"("Maximum"=w818) -> ()  [unwired: 2 in, 2 out]
        n465 = property on="Z Scan Length SP steps" class="DigNum (strict)"("Maximum"=w805) -> ()  [unwired: 2 in, 2 out]
        n466 = Divide(x=w791, y=w799) -> (x/y=w804:dbl)
        n467 = Divide(x=w783, y=w826) -> (x/y=w824:dbl)
        n468 = Divide(x=w787, y=w788) -> (x/y=w817:dbl)
        n469 = To Double Precision Float(number=w798) -> (double precision float=w790:dbl)
        n470 = To Double Precision Float(number=w830) -> (double precision float=w782:dbl)
        n471 = To Double Precision Float(number=w812) -> (double precision float=w786:dbl)
        n472 = property on="Z mm/rev" class="DigNum (strict)"() -> ("Value"=w801:dbl)  [unwired: 2 in, 2 out]
        n473 = property on="X mm/rev" class="DigNum (strict)"() -> ("Value"=w828:dbl)  [unwired: 2 in, 2 out]
        n474 = property on="Y mm/rev" class="DigNum (strict)"() -> ("Value"=w814:dbl)  [unwired: 2 in, 2 out]
        n475 = Multiply(x=w804, y=w801) -> (x*y=w796:dbl)
        n476 = Divide(x=w791, y=w790) -> (x/y=w789:dbl)
        n477 = Divide(x=w790, y=w799) -> (x/y=w797:dbl)
        n478 = Multiply(x=w828, y=w824) -> (x*y=w822:dbl)
        n479 = Divide(x=w783, y=w782) -> (x/y=w784:dbl)
        n480 = Divide(x=w782, y=w826) -> (x/y=w831:dbl)
        n481 = Multiply(x=w817, y=w814) -> (x*y=w810:dbl)
        n482 = Divide(x=w787, y=w786) -> (x/y=w785:dbl)
        n483 = Divide(x=w786, y=w788) -> (x/y=w811:dbl)
        n484 = Multiply(x=w801, y=w797) -> (x*y=w795:dbl)
        n485 = property on="X Scan length MV mm" class="DigNum (strict)"("Val(Sgnl)"=w822) -> ()  [unwired: 2 in, 2 out]
        n486 = Multiply(x=w831, y=w828) -> (x*y=w823:dbl)
        n487 = Multiply(x=w814, y=w811) -> (x*y=w809:dbl)
        n488 = property on="Z Scan length MV mm" class="DigNum (strict)"("Value"=w796) -> ()  [unwired: 2 in, 2 out]
        n489 = Absolute Value(x=w789) -> (abs(x)=→"Z Scan Duration":dbl)
        n490 = Absolute Value(x=w784) -> (abs(x)=→"X Scan Duration":dbl)
        n491 = property on="Y Scan length MV mm" class="DigNum (strict)"("Value"=w810) -> ()  [unwired: 2 in, 2 out]
        n492 = Absolute Value(x=w785) -> (abs(x)=→"Y Scan Duration":dbl)
        n493 = property on="Z Scan velocity MV mm/sec" class="DigNum (strict)"("Val(Sgnl)"=w795) -> ()  [unwired: 2 in, 2 out]
        n494 = property on="Y Scan velocity MV mm/sec" class="DigNum (strict)"("Val(Sgnl)"=w809) -> ()  [unwired: 2 in, 2 out]
        n495 = property on="X Scan velocity MV mm/sec" class="DigNum (strict)"("Value"=w823) -> ()  [unwired: 2 in, 2 out]
      }
      event "Y Move Set": Mouse Down {
        n496 = event-data() -> ()  [unwired: 1 in, 7 out]
        n497 = property on="Y steps/rev" class="DigNum (strict)"() -> ("Value"=w852:u32)  [unwired: 2 in, 2 out]
        n498 = property on="Y offset mm" class="DigNum (strict)"() -> ("Value"=w850:dbl)  [unwired: 2 in, 2 out]
        n499 = property on="Y Position SP mm" class="DigNum (strict)"() -> ("Value"=w849:dbl)  [unwired: 2 in, 2 out]
        n500 = property on="Y Velocity SP step/sec" class="DigNum (strict)"() -> ("Maximum"=w839:dbl)  [unwired: 2 in, 2 out]
        n501 = property on="Y Velocity SP step/sec" class="DigNum (strict)"() -> ("Minimum"=w838:dbl)  [unwired: 2 in, 2 out]
        n502 = Subtract(x=w849, y=w850) -> (x-y=w853:dbl)
        n503 = property on="Y Velocity SP mm/sec" class="DigNum (strict)"() -> ("Value"=w843:dbl)  [unwired: 2 in, 2 out]
        n504 = property on="Y mm/rev" class="DigNum (strict)"() -> ("Value"=w836:dbl)  [unwired: 2 in, 2 out]
        n505 = Divide(x=w853, y=w836) -> (x/y=w854:dbl)
        n506 = Divide(x=w843, y=w836) -> (x/y=w844:dbl)
        n507 = To Double Precision Float(number=w852) -> (double precision float=w837:dbl)
        n508 = Multiply(x=w854, y=w837) -> (x*y=w848:dbl)
        n509 = Multiply(x=w844, y=w837) -> (x*y=w841:dbl)
        n510 = property on="Y Step SP" class="DigNum (strict)"() -> ("Maximum"=w846:dbl)  [unwired: 2 in, 2 out]
        n511 = property on="Y Step SP" class="DigNum (strict)"() -> ("Minimum"=w845:dbl)  [unwired: 2 in, 2 out]
        n512 = In Range and Coerce(upper limit=w839, x=w841, lower limit=w838) -> (coerced(x)=w840:dbl)  [unwired: 1 out]
        n513 = To Long Integer(number=w840) -> (32bit integer=w842:i32)
        n514 = In Range and Coerce(upper limit=w846, x=w848, lower limit=w845) -> (coerced(x)=w847:dbl)  [unwired: 1 out]
        n515 = property on="Y Velocity SP step/sec" class="DigNum (strict)"("Val(Sgnl)"=w842) -> ()  [unwired: 2 in, 2 out]
        n516 = To Long Integer(number=w847) -> (32bit integer=w851:i32)
        n517 = property on="Y Step SP" class="DigNum (strict)"("Val(Sgnl)"=w851) -> ()  [unwired: 2 in, 2 out]
      }
      event "X Move Set": Mouse Down {
        n518 = event-data() -> ()  [unwired: 1 in, 7 out]
        n519 = property on="X steps/rev" class="DigNum (strict)"() -> ("Value"=w871:u32)  [unwired: 2 in, 2 out]
        n520 = property on="X offset mm" class="DigNum (strict)"() -> ("Value"=w869:dbl)  [unwired: 2 in, 2 out]
        n521 = property on="X Position SP mm" class="DigNum (strict)"() -> ("Value"=w868:dbl)  [unwired: 2 in, 2 out]
        n522 = property on="X Velocity SP step/sec" class="DigNum (strict)"() -> ("Maximum"=w858:dbl)  [unwired: 2 in, 2 out]
        n523 = property on="X Velocity SP step/sec" class="DigNum (strict)"() -> ("Minimum"=w857:dbl)  [unwired: 2 in, 2 out]
        n524 = Subtract(x=w868, y=w869) -> (x-y=w872:dbl)
        n525 = property on="X Velocity SP mm/sec" class="DigNum (strict)"() -> ("Value"=w862:dbl)  [unwired: 2 in, 2 out]
        n526 = property on="X mm/rev" class="DigNum (strict)"() -> ("Value"=w855:dbl)  [unwired: 2 in, 2 out]
        n527 = Divide(x=w872, y=w855) -> (x/y=w873:dbl)
        n528 = Divide(x=w862, y=w855) -> (x/y=w863:dbl)
        n529 = To Double Precision Float(number=w871) -> (double precision float=w856:dbl)
        n530 = Multiply(x=w873, y=w856) -> (x*y=w867:dbl)
        n531 = Multiply(x=w863, y=w856) -> (x*y=w860:dbl)
        n532 = property on="X Step SP" class="DigNum (strict)"() -> ("Maximum"=w865:dbl)  [unwired: 2 in, 2 out]
        n533 = property on="X Step SP" class="DigNum (strict)"() -> ("Minimum"=w864:dbl)  [unwired: 2 in, 2 out]
        n534 = In Range and Coerce(upper limit=w858, x=w860, lower limit=w857) -> (coerced(x)=w859:dbl)  [unwired: 1 out]
        n535 = To Long Integer(number=w859) -> (32bit integer=w861:i32)
        n536 = In Range and Coerce(upper limit=w865, x=w867, lower limit=w864) -> (coerced(x)=w866:dbl)  [unwired: 1 out]
        n537 = property on="X Velocity SP step/sec" class="DigNum (strict)"("Val(Sgnl)"=w861) -> ()  [unwired: 2 in, 2 out]
        n538 = To Long Integer(number=w866) -> (32bit integer=w870:i32)
        n539 = property on="X Step SP" class="DigNum (strict)"("Val(Sgnl)"=w870) -> ()  [unwired: 2 in, 2 out]
      }
      event "Z Move Set": Mouse Down {
        n540 = event-data() -> ()  [unwired: 1 in, 7 out]
        n541 = property on="Z steps/rev" class="DigNum (strict)"() -> ("Value"=w888:u32)  [unwired: 2 in, 2 out]
        n542 = property on="Z offset mm" class="DigNum (strict)"() -> ("Value"=w886:dbl)  [unwired: 2 in, 2 out]
        n543 = property on="Z Position SP mm" class="DigNum (strict)"() -> ("Value"=w885:dbl)  [unwired: 2 in, 2 out]
        n544 = property on="Z Velocity SP step/sec" class="DigNum (strict)"() -> ("Maximum"=w875:dbl)  [unwired: 2 in, 2 out]
        n545 = property on="Z Velocity SP step/sec" class="DigNum (strict)"() -> ("Minimum"=w874:dbl)  [unwired: 2 in, 2 out]
        n546 = Subtract(x=w885, y=w886) -> (x-y=w889:dbl)
        n547 = property on="Z Velocity SP mm/sec" class="DigNum (strict)"() -> ("Value"=w879:dbl)  [unwired: 2 in, 2 out]
        n548 = property on="Z mm/rev" class="DigNum (strict)"() -> ("Value"=w891:dbl)  [unwired: 2 in, 2 out]
        n549 = Divide(x=w889, y=w891) -> (x/y=w890:dbl)
        n550 = Divide(x=w879, y=w891) -> (x/y=w880:dbl)
        n551 = To Double Precision Float(number=w888) -> (double precision float=w892:dbl)
        n552 = Multiply(x=w890, y=w892) -> (x*y=w884:dbl)
        n553 = Multiply(x=w880, y=w892) -> (x*y=w877:dbl)
        n554 = property on="Z Step SP" class="DigNum (strict)"() -> ("Maximum"=w882:dbl)  [unwired: 2 in, 2 out]
        n555 = property on="Z Step SP" class="DigNum (strict)"() -> ("Minimum"=w881:dbl)  [unwired: 2 in, 2 out]
        n556 = In Range and Coerce(upper limit=w875, x=w877, lower limit=w874) -> (coerced(x)=w876:dbl)  [unwired: 1 out]
        n557 = To Long Integer(number=w876) -> (32bit integer=w878:i32)
        n558 = In Range and Coerce(upper limit=w882, x=w884, lower limit=w881) -> (coerced(x)=w883:dbl)  [unwired: 1 out]
        n559 = property on="Z Velocity SP step/sec" class="DigNum (strict)"("Val(Sgnl)"=w878) -> ()  [unwired: 2 in, 2 out]
        n560 = To Long Integer(number=w883) -> (32bit integer=w887:i32)
        n561 = property on="Z Step SP" class="DigNum (strict)"("Val(Sgnl)"=w887) -> ()  [unwired: 2 in, 2 out]
      }
      event "Y Scan set": Mouse Down {
        n562 = event-data() -> ()  [unwired: 1 in, 7 out]
        n563 = property on="Y steps/rev" class="DigNum (strict)"() -> ("Value"=w908:u32)  [unwired: 2 in, 2 out]
        n564 = To Double Precision Float(number=w908) -> (double precision float=w894:dbl)
        n565 = property on="Y mm/rev" class="DigNum (strict)"() -> ("Value"=w893:dbl)  [unwired: 2 in, 2 out]
        n566 = property on="Y Scan Length SP mm" class="DigNum (strict)"() -> ("Value"=w906:dbl)  [unwired: 2 in, 2 out]
        n567 = property on="Y Scan Velocity SP mm/sec" class="DigNum (strict)"() -> ("Value"=w900:dbl)  [unwired: 2 in, 2 out]
        n568 = property on="Y Scan Velocity SP steps/sec" class="DigNum (strict)"() -> ("Maximum"=w896:dbl)  [unwired: 2 in, 2 out]
        n569 = property on="Y Scan Velocity SP steps/sec" class="DigNum (strict)"() -> ("Minimum"=w895:dbl)  [unwired: 2 in, 2 out]
        n570 = Divide(x=w906, y=w893) -> (x/y=w909:dbl)
        n571 = Divide(x=w900, y=w893) -> (x/y=w901:dbl)
        n572 = Multiply(x=w909, y=w894) -> (x*y=w905:dbl)
        n573 = Multiply(x=w901, y=w894) -> (x*y=w898:dbl)
        n574 = property on="Y Step SP" class="DigNum (strict)"() -> ("Maximum"=w902:dbl)  [unwired: 2 in, 2 out]
        n575 = property on="Y Step SP" class="DigNum (strict)"() -> ("Minimum"=w903:dbl)  [unwired: 2 in, 2 out]
        n576 = In Range and Coerce(upper limit=w896, x=w898, lower limit=w895) -> (coerced(x)=w897:dbl)  [unwired: 1 out]
        n577 = To Long Integer(number=w897) -> (32bit integer=w899:i32)
        n578 = In Range and Coerce(upper limit=w902, x=w905, lower limit=w903) -> (coerced(x)=w904:dbl)  [unwired: 1 out]
        n579 = property on="Y Scan Velocity SP steps/sec" class="DigNum (strict)"("Val(Sgnl)"=w899) -> ()  [unwired: 2 in, 2 out]
        n580 = To Long Integer(number=w904) -> (32bit integer=w907:i32)
        n581 = property on="Y Scan Length SP steps" class="DigNum (strict)"("Val(Sgnl)"=w907) -> ()  [unwired: 2 in, 2 out]
      }
      event "X Scan set": Mouse Down {
        n582 = event-data() -> ()  [unwired: 1 in, 7 out]
        n583 = property on="X steps/rev" class="DigNum (strict)"() -> ("Value"=w925:u32)  [unwired: 2 in, 2 out]
        n584 = To Double Precision Float(number=w925) -> (double precision float=w911:dbl)
        n585 = property on="X mm/rev" class="DigNum (strict)"() -> ("Value"=w910:dbl)  [unwired: 2 in, 2 out]
        n586 = property on="X Scan Length SP mm" class="DigNum (strict)"() -> ("Value"=w923:dbl)  [unwired: 2 in, 2 out]
        n587 = property on="X Scan Velocity SP mm/sec" class="DigNum (strict)"() -> ("Value"=w917:dbl)  [unwired: 2 in, 2 out]
        n588 = property on="X Scan Velocity SP steps/sec" class="DigNum (strict)"() -> ("Maximum"=w913:dbl)  [unwired: 2 in, 2 out]
        n589 = property on="X Scan Velocity SP steps/sec" class="DigNum (strict)"() -> ("Minimum"=w912:dbl)  [unwired: 2 in, 2 out]
        n590 = Divide(x=w923, y=w910) -> (x/y=w926:dbl)
        n591 = Divide(x=w917, y=w910) -> (x/y=w918:dbl)
        n592 = Multiply(x=w926, y=w911) -> (x*y=w922:dbl)
        n593 = Multiply(x=w918, y=w911) -> (x*y=w915:dbl)
        n594 = property on="X Step SP" class="DigNum (strict)"() -> ("Maximum"=w919:dbl)  [unwired: 2 in, 2 out]
        n595 = property on="X Step SP" class="DigNum (strict)"() -> ("Minimum"=w920:dbl)  [unwired: 2 in, 2 out]
        n596 = In Range and Coerce(upper limit=w913, x=w915, lower limit=w912) -> (coerced(x)=w914:dbl)  [unwired: 1 out]
        n597 = To Long Integer(number=w914) -> (32bit integer=w916:i32)
        n598 = In Range and Coerce(upper limit=w919, x=w922, lower limit=w920) -> (coerced(x)=w921:dbl)  [unwired: 1 out]
        n599 = property on="X Scan Velocity SP steps/sec" class="DigNum (strict)"("Val(Sgnl)"=w916) -> ()  [unwired: 2 in, 2 out]
        n600 = To Long Integer(number=w921) -> (32bit integer=w924:i32)
        n601 = property on="X Scan Length SP steps" class="DigNum (strict)"("Val(Sgnl)"=w924) -> ()  [unwired: 2 in, 2 out]
      }
      event "Z Scan set": Mouse Down {
        n602 = event-data() -> ()  [unwired: 1 in, 7 out]
        n603 = property on="Z steps/rev" class="DigNum (strict)"() -> ("Value"=w942:u32)  [unwired: 2 in, 2 out]
        n604 = To Double Precision Float(number=w942) -> (double precision float=w928:dbl)
        n605 = property on="Z mm/rev" class="DigNum (strict)"() -> ("Value"=w927:dbl)  [unwired: 2 in, 2 out]
        n606 = property on="Z Scan Length SP mm" class="DigNum (strict)"() -> ("Value"=w940:dbl)  [unwired: 2 in, 2 out]
        n607 = property on="Z Scan Velocity SP mm/sec" class="DigNum (strict)"() -> ("Value"=w934:dbl)  [unwired: 2 in, 2 out]
        n608 = property on="Z Scan Velocity SP steps/sec" class="DigNum (strict)"() -> ("Maximum"=w930:dbl)  [unwired: 2 in, 2 out]
        n609 = property on="Z Scan Velocity SP steps/sec" class="DigNum (strict)"() -> ("Minimum"=w929:dbl)  [unwired: 2 in, 2 out]
        n610 = Divide(x=w940, y=w927) -> (x/y=w943:dbl)
        n611 = Divide(x=w934, y=w927) -> (x/y=w935:dbl)
        n612 = Multiply(x=w943, y=w928) -> (x*y=w939:dbl)
        n613 = Multiply(x=w935, y=w928) -> (x*y=w932:dbl)
        n614 = property on="Z Step SP" class="DigNum (strict)"() -> ("Maximum"=w936:dbl)  [unwired: 2 in, 2 out]
        n615 = property on="Z Step SP" class="DigNum (strict)"() -> ("Minimum"=w937:dbl)  [unwired: 2 in, 2 out]
        n616 = In Range and Coerce(upper limit=w930, x=w932, lower limit=w929) -> (coerced(x)=w931:dbl)  [unwired: 1 out]
        n617 = To Long Integer(number=w931) -> (32bit integer=w933:i32)
        n618 = In Range and Coerce(upper limit=w936, x=w939, lower limit=w937) -> (coerced(x)=w938:dbl)  [unwired: 1 out]
        n619 = property on="Z Scan Velocity SP steps/sec" class="DigNum (strict)"("Val(Sgnl)"=w933) -> ()  [unwired: 2 in, 2 out]
        n620 = To Long Integer(number=w938) -> (32bit integer=w941:i32)
        n621 = property on="Z Scan Length SP steps" class="DigNum (strict)"("Val(Sgnl)"=w941) -> ()  [unwired: 2 in, 2 out]
      }
      event "Y Go": Mouse Up {
        n622 = event-data() -> ()  [unwired: 1 in, 7 out]
        n623 = flat-sequence {
          tunnel: w950 -> [w960]
          tunnel: w951 -> [w961]
          tunnel: [w961] -> w947
          tunnel: [w960] -> w946
          tunnel: [w964] -> w949
          tunnel: [w963] -> w948
          tunnel: w947 -> [w966]
          tunnel: w946 -> [w965]
          tunnel: [w987] -> w953
          tunnel: [w982] -> w952
          tunnel: w949 -> [w986]
          tunnel: w948 -> [w985]
          tunnel: [w981] -> w945
          tunnel: [w998] -> w955
          tunnel: [w993] -> w954
          tunnel: w953 -> [w996]
          tunnel: w952 -> [w997]
          tunnel: w945 -> [w994]
          tunnel: [w994] -> w944
          tunnel: [w1001] -> w956
          tunnel: [w1004] -> w957
          tunnel: w955 -> [w1003]
          tunnel: w954 -> [w1002]
          tunnel: w944 -> [w1005]
          frame #0 {
            n624 = property on="Scan Go" class="Bool"("DisabledEnum"=T2."Disabled and Grayed Out" ("Disabled")) -> ()  [unwired: 2 in, 2 out]
            n625 = property on="Y Go" class="Bool"("DisabledEnum"=T2."Disabled and Grayed Out" ("Disabled")) -> ()  [unwired: 2 in, 2 out]
          }
          frame #1 {
            n626 = property on="Y Step SP" class="DigNum (strict)"() -> ("Value"=w974:i32)  [unwired: 2 in, 2 out]
            n627 = property on="Y Step PV" class="DigNum (strict)"() -> ("Value"=w973:i32)  [unwired: 2 in, 2 out]
            n628 = property on="Y Backlash" class="DigNum (strict)"() -> ("Value"=w962:i32)  [unwired: 2 in, 2 out]
            n629 = Subtract(x=w974, y=w973) -> (x-y=w972:i32)
            n630 = Sign(1:w962) -> (0:w970:i32)
            n631 = Sign(1:w972) -> (0:w971:i32)
            n632 = Multiply(x=w971, y=w970) -> (x*y=w969:i32)
            n633 = Equal?(x=w969, y=1) -> (x = y?=w967:bool)
            n634 = case shown="False" w967 {
              tunnel: w966 -> [w977 w979]
              tunnel: w965 -> [w976 w978]
              tunnel: [w976 w978] -> w964
              tunnel: [w977 w979] -> w963
              frame False {
                n635 = property on="Y Backlash corr" class="Bool (strict)"("Val(Sgnl)"=FALSE ("Value (Signaling)")) -> ()  [unwired: 2 in, 2 out]
              }
              frame True {
                n636 = property on="Y Backlash corr" class="Bool (strict)"("Val(Sgnl)"=TRUE ("Value (Signaling)")) -> ()  [unwired: 2 in, 2 out]
              }
            }
          }
          frame #2 {
            w981 = 0.1 ("Delay Time (s)")
            # "Velocity Setting"
            n637 = property on="Y Velocity SP step/sec" class="DigNum (strict)"() -> ("Value"=w990:i32)  [unwired: 2 in, 2 out]
            n638 = Number To Decimal String(number=w990) -> ()  [unwired: 1 in, 1 out]
            n639 = property on="Y steps/rev" class="DigNum (strict)"() -> ("Value"=w989:u32)  [unwired: 2 in, 2 out]
            n640 = Divide(x=w990, y=w989) -> (x/y=w991:dbl)
            n641 = Number To Fractional String(number=w991) -> (F-format string=w984:string)  [unwired: 3 in]
            n642 = call "Applied Send Command.vi"("error in (no error)"=w986, "Extra"=w984, "Command"=T1."Velocity Setting", "VISA resource name"=w985) -> ("error out"=w983:errorcluster, "VISA resource name out"=w987:refnum<visa-resource-name>)  [unwired: 3 in, 1 out]
            n643 = call "Time Delay22"("error in (no error)"=w983, "Delay Time (s)"=w981) -> ("error out"=w982:errorcluster)  [unwired: 9 in]
          }
          frame #3 {
            # "Move to Abs Position"
            n644 = property on="Y Step SP" class="DigNum (strict)"() -> ("Value"=w1000:i32)  [unwired: 2 in, 2 out]
            n645 = Number To Decimal String(number=w1000) -> (decimal integer string=w995:string)  [unwired: 1 in]
            n646 = call "Applied Send Command.vi"("error in (no error)"=w997, "Extra"=w995, "Command"=T1."Distance or Position", "VISA resource name"=w996) -> ("error out"=w992:errorcluster, "VISA resource name out"=w998:refnum<visa-resource-name>)  [unwired: 3 in, 1 out]
            n647 = call "Time Delay"("error in (no error)"=w992, "Delay Time (s)"=w994) -> ("error out"=w993:errorcluster)  [unwired: 9 in]
          }
          frame #4 {
            n648 = call "Applied Send Command.vi"("error in (no error)"=w1002, "Command"=T1."Feed to Position", "VISA resource name"=w1003) -> ("error out"=w1006:errorcluster, "VISA resource name out"=w1004:refnum<visa-resource-name>)  [unwired: 4 in, 1 out]
            n649 = call "Time Delay23"("error in (no error)"=w1006, "Delay Time (s)"=w1005) -> ("error out"=w1001:errorcluster)  [unwired: 9 in]
          }
        }
      }
      event "Z Go": Mouse Up {
        n650 = event-data() -> ()  [unwired: 1 in, 7 out]
        n651 = flat-sequence {
          tunnel: w1012 -> [w1024]
          tunnel: w1013 -> [w1025]
          tunnel: [w1025] -> w1015
          tunnel: [w1024] -> w1014
          tunnel: [w1028] -> w1017
          tunnel: [w1027] -> w1016
          tunnel: w1015 -> [w1030]
          tunnel: w1014 -> [w1029]
          tunnel: [w1048] -> w1019
          tunnel: [w1046] -> w1018
          tunnel: w1017 -> [w1049]
          tunnel: w1016 -> [w1050]
          tunnel: [w1045] -> w1009
          tunnel: [w1059] -> w1021
          tunnel: [w1058] -> w1020
          tunnel: w1019 -> [w1060]
          tunnel: w1018 -> [w1062]
          tunnel: w1009 -> [w1056]
          tunnel: [w1056] -> w1008
          tunnel: [w1071] -> w1011
          tunnel: [w1067] -> w1010
          tunnel: w1021 -> [w1068]
          tunnel: w1020 -> [w1065]
          tunnel: w1008 -> [w1070]
          frame #0 {
            n652 = property on="Scan Go" class="Bool"("DisabledEnum"=T2."Disabled and Grayed Out" ("Disabled")) -> ()  [unwired: 2 in, 2 out]
            n653 = property on="Z Go" class="Bool"("DisabledEnum"=T2."Disabled and Grayed Out" ("Disabled")) -> ()  [unwired: 2 in, 2 out]
          }
          frame #1 {
            n654 = property on="Z Step SP" class="DigNum (strict)"() -> ("Value"=w1038:i32)  [unwired: 2 in, 2 out]
            n655 = property on="Z Step PV" class="DigNum (strict)"() -> ("Value"=w1037:i32)  [unwired: 2 in, 2 out]
            n656 = property on="Z Backlash" class="DigNum (strict)"() -> ("Value"=w1026:i32)  [unwired: 2 in, 2 out]
            n657 = Subtract(x=w1038, y=w1037) -> (x-y=w1036:i32)
            n658 = Sign(1:w1026) -> (0:w1034:i32)
            n659 = Sign(1:w1036) -> (0:w1035:i32)
            n660 = Multiply(x=w1035, y=w1034) -> (x*y=w1033:i32)
            n661 = Equal?(x=w1033, y=1) -> (x = y?=w1031:bool)
            n662 = case shown="True" w1031 {
              tunnel: w1030 -> [w1041 w1043]
              tunnel: w1029 -> [w1040 w1042]
              tunnel: [w1040 w1042] -> w1028
              tunnel: [w1041 w1043] -> w1027
              frame False {
                n663 = property on="Z Backlash corr" class="Bool (strict)"("Val(Sgnl)"=FALSE ("Value (Signaling)")) -> ()  [unwired: 2 in, 2 out]
              }
              frame True {
                n664 = property on="Z Backlash corr" class="Bool (strict)"("Val(Sgnl)"=TRUE ("Value (Signaling)")) -> ()  [unwired: 2 in, 2 out]
              }
            }
          }
          frame #2 {
            w1045 = 0.1 ("Delay Time (s)")
            n665 = property on="Z Velocity SP step/sec" class="DigNum (strict)"() -> ("Value"=w1052:i32)  [unwired: 2 in, 2 out]
            n666 = property on="Z steps/rev" class="DigNum (strict)"() -> ("Value"=w1051:u32)  [unwired: 2 in, 2 out]
            n667 = Divide(x=w1052, y=w1051) -> (x/y=w1053:dbl)
            n668 = Number To Fractional String(number=w1053) -> (F-format string=w1054:string)  [unwired: 3 in]
            n669 = call "Applied Send Command.vi"("error in (no error)"=w1049, "Extra"=w1054, "Command"=T1."Velocity Setting", "VISA resource name"=w1050) -> ("error out"=w1047:errorcluster, "VISA resource name out"=w1048:refnum<visa-resource-name>)  [unwired: 3 in, 1 out]
            n670 = call "Time Delay52"("error in (no error)"=w1047, "Delay Time (s)"=w1045) -> ("error out"=w1046:errorcluster)  [unwired: 9 in]
          }
          frame #3 {
            # "Move to Abs Position"
            n671 = property on="Z Step SP" class="DigNum (strict)"() -> ("Value"=w1064:i32)  [unwired: 2 in, 2 out]
            n672 = Number To Decimal String(number=w1064) -> (decimal integer string=w1061:string)  [unwired: 1 in]
            n673 = call "Applied Send Command.vi"("error in (no error)"=w1062, "Extra"=w1061, "Command"=T1."Distance or Position", "VISA resource name"=w1060) -> ("error out"=w1057:errorcluster, "VISA resource name out"=w1059:refnum<visa-resource-name>)  [unwired: 3 in, 1 out]
            n674 = call "Time Delay51"("error in (no error)"=w1057, "Delay Time (s)"=w1056) -> ("error out"=w1058:errorcluster)  [unwired: 9 in]
          }
          frame #4 {
            n675 = call "Applied Send Command.vi"("error in (no error)"=w1065, "Command"=T1."Feed to Position", "VISA resource name"=w1068) -> ("error out"=w1066:errorcluster, "VISA resource name out"=w1067:refnum<visa-resource-name>)  [unwired: 4 in, 1 out]
            n676 = call "Time Delay28"("error in (no error)"=w1066, "Delay Time (s)"=w1070) -> ("error out"=w1071:errorcluster)  [unwired: 9 in]
          }
        }
      }
      event "X Go": Mouse Up {
        n677 = event-data() -> ()  [unwired: 1 in, 7 out]
        n678 = flat-sequence {
          tunnel: [w1087] -> w1083
          tunnel: [w1086] -> w1082
          tunnel: w1081 -> [w1087]
          tunnel: w1080 -> [w1086]
          tunnel: [w1092] -> w1085
          tunnel: [w1091] -> w1084
          tunnel: w1083 -> [w1094]
          tunnel: w1082 -> [w1093]
          tunnel: [w1113] -> w1077
          tunnel: [w1110] -> w1075
          tunnel: w1085 -> [w1114]
          tunnel: w1084 -> [w1115]
          tunnel: [w1109] -> w1073
          tunnel: w1077 -> [w1122]
          tunnel: [w1121] -> w1076
          tunnel: w1075 -> [w1123]
          tunnel: [w1124] -> w1074
          tunnel: w1073 -> [w1120]
          tunnel: [w1120] -> w1072
          tunnel: w1076 -> [w1134]
          tunnel: w1074 -> [w1133]
          tunnel: [w1132] -> w1079
          tunnel: [w1131] -> w1078
          tunnel: w1072 -> [w1129]
          frame #0 {
            n679 = property on="Scan Go" class="Bool"("DisabledEnum"=T2."Disabled and Grayed Out" ("Disabled")) -> ()  [unwired: 2 in, 2 out]
            n680 = property on="X Go" class="Bool"("DisabledEnum"=T2."Disabled and Grayed Out" ("Disabled")) -> ()  [unwired: 2 in, 2 out]
          }
          frame #1 {
            n681 = property on="X Step SP" class="DigNum (strict)"() -> ("Value"=w1102:i32)  [unwired: 2 in, 2 out]
            n682 = property on="X Step PV" class="DigNum (strict)"() -> ("Value"=w1101:i32)  [unwired: 2 in, 2 out]
            n683 = property on="X Backlash" class="DigNum (strict)"() -> ("Value"=w1090:i32)  [unwired: 2 in, 2 out]
            n684 = Subtract(x=w1102, y=w1101) -> (x-y=w1100:i32)
            n685 = Sign(1:w1090) -> (0:w1098:i32)
            n686 = Sign(1:w1100) -> (0:w1099:i32)
            n687 = Multiply(x=w1099, y=w1098) -> (x*y=w1097:i32)
            n688 = Equal?(x=w1097, y=1) -> (x = y?=w1095:bool)
            n689 = case shown="True" w1095 {
              tunnel: w1094 -> [w1105 w1107]
              tunnel: w1093 -> [w1104 w1106]
              tunnel: [w1104 w1106] -> w1092
              tunnel: [w1105 w1107] -> w1091
              frame False {
                n690 = property on="X Backlash corr" class="Bool (strict)"("Val(Sgnl)"=FALSE ("Value (Signaling)")) -> ()  [unwired: 2 in, 2 out]
              }
              frame True {
                n691 = property on="X Backlash corr" class="Bool (strict)"("Val(Sgnl)"=TRUE ("Value (Signaling)")) -> ()  [unwired: 2 in, 2 out]
              }
            }
          }
          frame #2 {
            w1109 = 0.1 ("Delay Time (s)")
            n692 = property on="X Velocity SP step/sec" class="DigNum (strict)"() -> ("Value"=w1112:i32)  [unwired: 2 in, 2 out]
            n693 = property on="X steps/rev" class="DigNum (strict)"() -> ("Value"=w1116:u32)  [unwired: 2 in, 2 out]
            n694 = Divide(x=w1112, y=w1116) -> (x/y=w1117:dbl)
            n695 = Number To Fractional String(number=w1117) -> (F-format string=w1118:string)  [unwired: 3 in]
            n696 = call "Applied Send Command.vi"("error in (no error)"=w1114, "Extra"=w1118, "Command"=T1."Velocity Setting", "VISA resource name"=w1115) -> ("error out"=w1111:errorcluster, "VISA resource name out"=w1113:refnum<visa-resource-name>)  [unwired: 3 in, 1 out]
            n697 = call "Time Delay14"("error in (no error)"=w1111, "Delay Time (s)"=w1109) -> ("error out"=w1110:errorcluster)  [unwired: 9 in]
          }
          frame #3 {
            # "Distance/Position"
            n698 = property on="X Step SP" class="DigNum (strict)"() -> ("Value"=w1125:i32)  [unwired: 2 in, 2 out]
            n699 = Number To Decimal String(number=w1125) -> (decimal integer string=w1127:string)  [unwired: 1 in]
            n700 = call "Applied Send Command.vi"("error in (no error)"=w1123, "Extra"=w1127, "Command"=T1."Distance or Position", "VISA resource name"=w1122) -> ("error out"=w1126:errorcluster, "VISA resource name out"=w1121:refnum<visa-resource-name>)  [unwired: 3 in, 1 out]
            n701 = call "Time Delay31"("error in (no error)"=w1126, "Delay Time (s)"=w1120) -> ("error out"=w1124:errorcluster)  [unwired: 9 in]
          }
          frame #4 {
            # "Feed to Position"
            n702 = call "Applied Send Command.vi"("error in (no error)"=w1133, "Command"=T1."Feed to Position", "VISA resource name"=w1134) -> ("error out"=w1130:errorcluster, "VISA resource name out"=w1132:refnum<visa-resource-name>)  [unwired: 4 in, 1 out]
            n703 = call "Time Delay15"("error in (no error)"=w1130, "Delay Time (s)"=w1129) -> ("error out"=w1131:errorcluster)  [unwired: 9 in]
          }
        }
      }
      event "X Scan OK": Mouse Up {
        n704 = event-data() -> ()  [unwired: 1 in, 7 out]
        n705 = flat-sequence {
          tunnel: [w1151] -> w1143
          tunnel: [w1162] -> w1142
          tunnel: w1141 -> [w1159]
          tunnel: w1140 -> [w1158]
          tunnel: w1143 -> [w1169]
          tunnel: w1142 -> [w1168]
          tunnel: [w1169] -> w1137
          tunnel: [w1168] -> w1136
          tunnel: [w1171] -> w1138
          tunnel: [w1172] -> w1139
          tunnel: w1137 -> [w1172]
          tunnel: w1136 -> [w1171]
          frame #0 {
            # "VELOCITY"
            n706 = property on="X steps/rev" class="DigNum (strict)"() -> ("Value"=w1144:u32)  [unwired: 2 in, 2 out]
            n707 = property on="X Scan Velocity SP steps/sec" class="DigNum (strict)"() -> ("Value"=w1145:i32)  [unwired: 2 in, 2 out]
            n708 = Divide(x=w1145, y=w1144) -> (x/y=w1146:dbl)
            n709 = Number To Fractional String(number=w1146) -> (F-format string=w1160:string)  [unwired: 3 in]
            n710 = call "Applied Send Command.vi"("error in (no error)"=w1158, "Extra"=w1160, "Command"=T1."Velocity Setting", "VISA resource name"=w1159) -> ("error out"=w1147:errorcluster, "VISA resource name out"=w1148:refnum<visa-resource-name>)  [unwired: 3 in, 1 out]
            n711 = call "Time Delay9"("error in (no error)"=w1147) -> ("error out"=w1149:errorcluster)  [unwired: 10 in]
            n712 = call "Applied Send Command.vi"("error in (no error)"=w1149, "Extra"="", "Command"=T1."Velocity Setting", "VISA resource name"=w1148) -> ("error out"=w1150:errorcluster, "read buffer"=w1155:string, "VISA resource name out"=w1151:refnum<visa-resource-name>)  [unwired: 3 in]
            n713 = call "Time Delay10"("error in (no error)"=w1150) -> ("error out"=w1162:errorcluster)  [unwired: 10 in]
            n714 = Fract/Exp String To Number(string=w1155, offset=3) -> (number=w1153:dbl)  [unwired: 2 in, 1 out]
            n715 = Multiply(x=w1153, y=w1144) -> (x*y=w1152:dbl)
            n716 = property on="X velocity PV step/sec" class="DigNum (strict)"("Val(Sgnl)"=w1152) -> ()  [unwired: 2 in, 2 out]
          }
          frame #1 {
            n717 = property on="X Scan" class="Bool (strict)"("Val(Sgnl)"=TRUE ("Slew Ready 2")) -> ()  [unwired: 2 in, 2 out]
            n718 = property on="Scan Cancel" class="Bool"("DisabledEnum"=T2."Enabled" ("Disabled")) -> ()  [unwired: 2 in, 2 out]
            n719 = property on="Scan Go" class="Bool"("DisabledEnum"=T2."Enabled" ("Disabled")) -> ()  [unwired: 2 in, 2 out]
            n720 = property on="X Scan Length SP steps" class="DigNum (strict)"("DisabledEnum"=T2."Disabled and Grayed Out" ("Disabled")) -> ()  [unwired: 2 in, 2 out]
            n721 = property on="X Scan Velocity SP steps/sec" class="DigNum (strict)"("DisabledEnum"=T2."Disabled and Grayed Out" ("Disabled")) -> ()  [unwired: 2 in, 2 out]
          }
          frame #2 {
            n722 = property on="X Go" class="Bool"("DisabledEnum"=T2."Disabled and Grayed Out" ("Disabled")) -> ()  [unwired: 2 in, 2 out]
          }
        }
      }
      event "Y Scan OK": Mouse Up {
        n723 = event-data() -> ()  [unwired: 1 in, 7 out]
        n724 = flat-sequence {
          tunnel: w1180 -> [w1192]
          tunnel: w1179 -> [w1193]
          tunnel: [w1183] -> w1177
          tunnel: [w1199] -> w1176
          tunnel: w1177 -> [w1206]
          tunnel: w1176 -> [w1205]
          tunnel: [w1206] -> w1174
          tunnel: [w1205] -> w1173
          tunnel: [w1208] -> w1178
          tunnel: [w1209] -> w1175
          tunnel: w1174 -> [w1209]
          tunnel: w1173 -> [w1208]
          frame #0 {
            # "VELOCITY"
            n725 = property on="Y Scan Velocity SP steps/sec" class="DigNum (strict)"() -> ("Value"=w1195:i32)  [unwired: 2 in, 2 out]
            n726 = property on="Y steps/rev" class="DigNum (strict)"() -> ("Value"=w1186:u32)  [unwired: 2 in, 2 out]
            n727 = Divide(x=w1195, y=w1186) -> (x/y=w1196:dbl)
            n728 = Number To Fractional String(number=w1196) -> (F-format string=w1197:string)  [unwired: 3 in]
            n729 = call "Applied Send Command.vi"("error in (no error)"=w1192, "Extra"=w1197, "Command"=T1."Velocity Setting", "VISA resource name"=w1193) -> ("error out"=w1194:errorcluster, "VISA resource name out"=w1184:refnum<visa-resource-name>)  [unwired: 3 in, 1 out]
            n730 = call "Time Delay5"("error in (no error)"=w1194) -> ("error out"=w1185:errorcluster)  [unwired: 10 in]
            n731 = call "Applied Send Command.vi"("error in (no error)"=w1185, "Extra"="", "Command"=T1."Velocity Setting", "VISA resource name"=w1184) -> ("error out"=w1182:errorcluster, "read buffer"=w1189:string, "VISA resource name out"=w1183:refnum<visa-resource-name>)  [unwired: 3 in]
            n732 = Fract/Exp String To Number(string=w1189, offset=3) -> (number=w1188:dbl)  [unwired: 2 in, 1 out]
            n733 = call "Time Delay6"("error in (no error)"=w1182) -> ("error out"=w1199:errorcluster)  [unwired: 10 in]
            n734 = Multiply(x=w1188, y=w1186) -> (x*y=w1187:dbl)
            n735 = property on="Y velocity PV step/sec" class="DigNum (strict)"("Val(Sgnl)"=w1187) -> ()  [unwired: 2 in, 2 out]
          }
          frame #1 {
            n736 = property on="Y Scan" class="Bool (strict)"("Val(Sgnl)"=TRUE ("Slew Ready 2")) -> ()  [unwired: 2 in, 2 out]
            n737 = property on="Scan Cancel" class="Bool"("DisabledEnum"=T2."Enabled" ("Disabled")) -> ()  [unwired: 2 in, 2 out]
            n738 = property on="Scan Go" class="Bool"("DisabledEnum"=T2."Enabled" ("Disabled")) -> ()  [unwired: 2 in, 2 out]
            n739 = property on="Y Scan Length SP steps" class="DigNum (strict)"("DisabledEnum"=T2."Disabled and Grayed Out" ("Disabled")) -> ()  [unwired: 2 in, 2 out]
            n740 = property on="Y Scan Velocity SP steps/sec" class="DigNum (strict)"("DisabledEnum"=T2."Disabled and Grayed Out" ("Disabled")) -> ()  [unwired: 2 in, 2 out]
          }
          frame #2 {
            n741 = property on="Y Go" class="Bool"("DisabledEnum"=T2."Disabled and Grayed Out" ("Disabled")) -> ()  [unwired: 2 in, 2 out]
          }
        }
      }
      event "Z Scan OK": Mouse Up {
        n742 = event-data() -> ()  [unwired: 1 in, 7 out]
        n743 = flat-sequence {
          tunnel: [w1222] -> w1217
          tunnel: [w1236] -> w1216
          tunnel: w1213 -> [w1218]
          tunnel: w1212 -> [w1219]
          tunnel: w1217 -> [w1243]
          tunnel: w1216 -> [w1242]
          tunnel: [w1243] -> w1215
          tunnel: [w1242] -> w1214
          tunnel: [w1245] -> w1211
          tunnel: [w1246] -> w1210
          tunnel: w1215 -> [w1246]
          tunnel: w1214 -> [w1245]
          frame #0 {
            # "VELOCITY"
            n744 = property on="Z Scan Velocity SP steps/sec" class="DigNum (strict)"() -> ("Value"=w1232:i32)  [unwired: 2 in, 2 out]
            n745 = property on="Z steps/rev" class="DigNum (strict)"() -> ("Value"=w1225:u32)  [unwired: 2 in, 2 out]
            n746 = Divide(x=w1232, y=w1225) -> (x/y=w1233:dbl)
            n747 = Number To Fractional String(number=w1233) -> (F-format string=w1234:string)  [unwired: 3 in]
            n748 = call "Applied Send Command.vi"("error in (no error)"=w1219, "Extra"=w1234, "Command"=T1."Velocity Setting", "VISA resource name"=w1218) -> ("error out"=w1231:errorcluster, "VISA resource name out"=w1221:refnum<visa-resource-name>)  [unwired: 3 in, 1 out]
            n749 = call "Time Delay24"("error in (no error)"=w1231) -> ("error out"=w1220:errorcluster)  [unwired: 10 in]
            n750 = call "Applied Send Command.vi"("error in (no error)"=w1220, "Extra"="", "Command"=T1."Velocity Setting", "VISA resource name"=w1221) -> ("error out"=w1223:errorcluster, "read buffer"=w1228:string, "VISA resource name out"=w1222:refnum<visa-resource-name>)  [unwired: 3 in]
            n751 = call "Time Delay25"("error in (no error)"=w1223) -> ("error out"=w1236:errorcluster)  [unwired: 10 in]
            n752 = Fract/Exp String To Number(string=w1228, offset=3) -> (number=w1227:dbl)  [unwired: 2 in, 1 out]
            n753 = Multiply(x=w1227, y=w1225) -> (x*y=w1224:dbl)
            n754 = property on="Z  velocity PV step/sec" class="DigNum (strict)"("Val(Sgnl)"=w1224) -> ()  [unwired: 2 in, 2 out]
          }
          frame #1 {
            n755 = property on="Z Scan" class="Bool (strict)"("Val(Sgnl)"=TRUE ("Slew Ready 2")) -> ()  [unwired: 2 in, 2 out]
            n756 = property on="Scan Cancel" class="Bool"("DisabledEnum"=T2."Enabled" ("Disabled")) -> ()  [unwired: 2 in, 2 out]
            n757 = property on="Scan Go" class="Bool"("DisabledEnum"=T2."Enabled" ("Disabled")) -> ()  [unwired: 2 in, 2 out]
            n758 = property on="Z Scan Length SP steps" class="DigNum (strict)"("DisabledEnum"=T2."Disabled and Grayed Out" ("Disabled")) -> ()  [unwired: 2 in, 2 out]
            n759 = property on="Z Scan Velocity SP steps/sec" class="DigNum (strict)"("DisabledEnum"=T2."Disabled and Grayed Out" ("Disabled")) -> ()  [unwired: 2 in, 2 out]
          }
          frame #2 {
            n760 = property on="Z Go" class="Bool"("DisabledEnum"=T2."Disabled and Grayed Out" ("Disabled")) -> ()  [unwired: 2 in, 2 out]
          }
        }
      }
      event Application Instance Close? {
        n761 = event-data() -> ()  [unwired: 1 in, 4 out]
        n762 = event-data() -> ()  [unwired: 3 in, 1 out]
      }
      event "Stop": Mouse Down {
        n763 = event-data() -> ()  [unwired: 1 in, 7 out]
        n764 = flat-sequence {
          tunnel: [w1268] -> w1256
          tunnel: [w1267] -> w1255
          tunnel: w1254 -> [w1269]
          tunnel: w1253 -> [w1266]
          frame #0 {
            n765 = call "Applied Send Command.vi"("error in (no error)"=w1266, "Command"=T1."Stop", "VISA resource name"=w1269) -> ("error out"=w1267:errorcluster, "VISA resource name out"=w1268:refnum<visa-resource-name>)  [unwired: 4 in, 1 out]
          }
        }
        n766 = flat-sequence {
          tunnel: w1260 -> [w1272]
          tunnel: w1259 -> [w1271]
          tunnel: [w1273] -> w1258
          tunnel: [w1274] -> w1257
          frame #0 {
            n767 = call "Applied Send Command.vi"("error in (no error)"=w1271, "Command"=T1."Stop", "VISA resource name"=w1272) -> ("error out"=w1274:errorcluster, "VISA resource name out"=w1273:refnum<visa-resource-name>)  [unwired: 4 in, 1 out]
          }
        }
        n768 = flat-sequence {
          tunnel: [w1263] -> w1250
          tunnel: [w1264] -> w1249
          tunnel: w1252 -> [w1261]
          tunnel: w1251 -> [w1262]
          frame #0 {
            n769 = call "Applied Send Command.vi"("error in (no error)"=w1262, "Command"=T1."Stop", "VISA resource name"=w1261) -> ("error out"=w1264:errorcluster, "VISA resource name out"=w1263:refnum<visa-resource-name>)  [unwired: 4 in, 1 out]
          }
        }
      }
      event "Scan Cancel": Mouse Down {
        n770 = event-data() -> ()  [unwired: 1 in, 7 out]
        n771 = flat-sequence {
          tunnel: w1285 -> [w1310]
          tunnel: w1284 -> [w1309]
          tunnel: [w1312] -> w1287
          tunnel: [w1311] -> w1286
          tunnel: [w1320] -> w1282
          tunnel: [w1321] -> w1283
          tunnel: w1287 -> [w1321]
          tunnel: w1286 -> [w1320]
          frame #0 {
            n772 = call "Applied Send Command.vi"("error in (no error)"=w1309, "Command"=T1."Stop", "VISA resource name"=w1310) -> ("error out"=w1311:errorcluster, "VISA resource name out"=w1312:refnum<visa-resource-name>)  [unwired: 4 in, 1 out]
          }
          frame #1 {
            n773 = property on="X Scan" class="Bool (strict)"("Value"=FALSE ("Slew Ready")) -> ()  [unwired: 2 in, 2 out]
            n774 = property on="X Scan set" class="Bool"("DisabledEnum"=T2."Enabled" ("Disabled")) -> ()  [unwired: 2 in, 2 out]
            n775 = property on="X Scan Velocity SP steps/sec" class="DigNum (strict)"("DisabledEnum"=T2."Enabled" ("Disabled")) -> ()  [unwired: 2 in, 2 out]
            n776 = property on="X Scan Length SP steps" class="DigNum (strict)"("DisabledEnum"=T2."Enabled" ("Disabled")) -> ()  [unwired: 2 in, 2 out]
            n777 = property on="X Go" class="Bool"("DisabledEnum"=T2."Enabled" ("Disabled")) -> ()  [unwired: 2 in, 2 out]
            n778 = property on="X Scan OK" class="Bool"("DisabledEnum"=T2."Enabled" ("Disabled")) -> ()  [unwired: 2 in, 2 out]
          }
        }
        n779 = flat-sequence {
          tunnel: w1293 -> [w1323]
          tunnel: w1292 -> [w1322]
          tunnel: [w1325] -> w1289
          tunnel: [w1324] -> w1288
          tunnel: [w1333] -> w1294
          tunnel: [w1334] -> w1295
          tunnel: w1289 -> [w1334]
          tunnel: w1288 -> [w1333]
          frame #0 {
            n780 = call "Applied Send Command.vi"("error in (no error)"=w1322, "Command"=T1."Stop", "VISA resource name"=w1323) -> ("error out"=w1324:errorcluster, "VISA resource name out"=w1325:refnum<visa-resource-name>)  [unwired: 4 in, 1 out]
          }
          frame #1 {
            n781 = property on="Y Scan" class="Bool (strict)"("Value"=FALSE ("Slew Ready")) -> ()  [unwired: 2 in, 2 out]
            n782 = property on="Y Go" class="Bool"("DisabledEnum"=T2."Enabled" ("Disabled")) -> ()  [unwired: 2 in, 2 out]
            n783 = property on="Y Scan Velocity SP steps/sec" class="DigNum (strict)"("DisabledEnum"=T2."Enabled" ("Disabled")) -> ()  [unwired: 2 in, 2 out]
            n784 = property on="Y Scan set" class="Bool"("DisabledEnum"=T2."Enabled" ("Disabled")) -> ()  [unwired: 2 in, 2 out]
            n785 = property on="Y Scan OK" class="Bool"("DisabledEnum"=T2."Enabled" ("Disabled")) -> ()  [unwired: 2 in, 2 out]
            n786 = property on="Y Scan Length SP steps" class="DigNum (strict)"("DisabledEnum"=T2."Enabled" ("Disabled")) -> ()  [unwired: 2 in, 2 out]
          }
        }
        n787 = flat-sequence {
          tunnel: [w1299] -> w1281
          tunnel: [w1298] -> w1280
          tunnel: w1279 -> [w1297]
          tunnel: w1278 -> [w1296]
          tunnel: [w1307] -> w1276
          tunnel: [w1308] -> w1277
          tunnel: w1281 -> [w1308]
          tunnel: w1280 -> [w1307]
          frame #0 {
            n788 = call "Applied Send Command.vi"("error in (no error)"=w1296, "Command"=T1."Stop", "VISA resource name"=w1297) -> ("error out"=w1298:errorcluster, "VISA resource name out"=w1299:refnum<visa-resource-name>)  [unwired: 4 in, 1 out]
          }
          frame #1 {
            n789 = property on="Z Scan" class="Bool (strict)"("Value"=FALSE ("Slew Ready")) -> ()  [unwired: 2 in, 2 out]
            n790 = property on="Z Scan set" class="Bool"("DisabledEnum"=T2."Enabled" ("Disabled")) -> ()  [unwired: 2 in, 2 out]
            n791 = property on="Z Scan Velocity SP steps/sec" class="DigNum (strict)"("DisabledEnum"=T2."Enabled" ("Disabled")) -> ()  [unwired: 2 in, 2 out]
            n792 = property on="Z Scan Length SP steps" class="DigNum (strict)"("DisabledEnum"=T2."Enabled" ("Disabled")) -> ()  [unwired: 2 in, 2 out]
            n793 = property on="Z Go" class="Bool"("DisabledEnum"=T2."Enabled" ("Disabled")) -> ()  [unwired: 2 in, 2 out]
            n794 = property on="Z Scan OK" class="Bool"("DisabledEnum"=T2."Enabled" ("Disabled")) -> ()  [unwired: 2 in, 2 out]
          }
        }
        n795 = property on="Scan Go" class="Bool"("DisabledEnum"=T2."Disabled and Grayed Out" ("Disabled")) -> ()  [unwired: 2 in, 2 out]
        n796 = property on="Scan Cancel" class="Bool"("DisabledEnum"=T2."Disabled and Grayed Out" ("Disabled")) -> ()  [unwired: 2 in, 2 out]
      }
      event "Scan Go": Mouse Up {
        n797 = event-data() -> ()  [unwired: 1 in, 7 out]
        n798 = flat-sequence {
          tunnel: w1361 -> [w1375]
          tunnel: w1360 -> [w1376]
          tunnel: w1359 -> [w1373]
          tunnel: w1358 -> [w1374]
          tunnel: w1357 -> [w1372]
          tunnel: w1356 -> [w1371]
          tunnel: [w1370] -> w1349
          tunnel: [w1369] -> w1347
          tunnel: [w1368] -> w1345
          tunnel: [w1367] -> w1343
          tunnel: [w1366] -> w1341
          tunnel: [w1365] -> w1339
          tunnel: [w1364] -> w1337
          tunnel: [w1363] -> w1336
          tunnel: [w1362] -> w1335
          tunnel: w1349 -> [w1418]
          tunnel: [w1417] -> w1348
          tunnel: w1347 -> [w1416]
          tunnel: [w1415] -> w1346
          tunnel: w1345 -> [w1414]
          tunnel: [w1413] -> w1344
          tunnel: w1343 -> [w1412]
          tunnel: [w1411] -> w1342
          tunnel: w1341 -> [w1410]
          tunnel: [w1409] -> w1340
          tunnel: w1339 -> [w1407]
          tunnel: [w1408] -> w1338
          tunnel: w1337 -> [w1406]
          tunnel: w1336 -> [w1405]
          tunnel: w1335 -> [w1404]
          tunnel: [w1444] -> w1355
          tunnel: [w1443] -> w1354
          tunnel: [w1442] -> w1353
          tunnel: [w1441] -> w1352
          tunnel: [w1446] -> w1351
          tunnel: [w1445] -> w1350
          tunnel: w1348 -> [w1446]
          tunnel: w1346 -> [w1445]
          tunnel: w1344 -> [w1444]
          tunnel: w1342 -> [w1443]
          tunnel: w1340 -> [w1442]
          tunnel: w1338 -> [w1441]
          frame #0 {
            n799 = property on="X Scan" class="Bool (strict)"() -> ("Value"=w1362:bool)  [unwired: 2 in, 2 out]
            n800 = property on="Y Scan" class="Bool (strict)"() -> ("Value"=w1363:bool)  [unwired: 2 in, 2 out]
            n801 = property on="Z Scan" class="Bool (strict)"() -> ("Value"=w1364:bool)  [unwired: 2 in, 2 out]
            n802 = case shown="True" w1362 {
              tunnel: w1376 -> [w1387 w1391]
              tunnel: [w1387 w1390] -> w1369
              tunnel: w1375 -> [w1386 w1389]
              tunnel: [w1386 w1388] -> w1370
              frame False {
              }
              frame True {
                n803 = property on="X Scan Length SP steps" class="DigNum (strict)"() -> ("Value"=w1392:i32)  [unwired: 2 in, 2 out]
                n804 = Number To Decimal String(number=w1392) -> (decimal integer string=w1393:string)  [unwired: 1 in]
                n805 = call "Applied Send Command.vi"("error in (no error)"=w1391, "Extra"=w1393, "Command"=T1."Distance or Position", "VISA resource name"=w1389) -> ("error out"=w1390:errorcluster, "VISA resource name out"=w1388:refnum<visa-resource-name>)  [unwired: 3 in, 1 out]
              }
            }
            n806 = case shown="True" w1363 {
              tunnel: w1373 -> [w1396 w1401]
              tunnel: w1374 -> [w1395 w1400]
              tunnel: [w1395 w1397] -> w1367
              tunnel: [w1396 w1398] -> w1368
              frame False {
              }
              frame True {
                n807 = property on="Y Scan Length SP steps" class="DigNum (strict)"() -> ("Value"=w1399:i32)  [unwired: 2 in, 2 out]
                n808 = Number To Decimal String(number=w1399) -> (decimal integer string=w1402:string)  [unwired: 1 in]
                n809 = call "Applied Send Command.vi"("error in (no error)"=w1400, "Extra"=w1402, "Command"=T1."Distance or Position", "VISA resource name"=w1401) -> ("error out"=w1397:errorcluster, "VISA resource name out"=w1398:refnum<visa-resource-name>)  [unwired: 3 in, 1 out]
              }
            }
            n810 = case shown="True" w1364 {
              tunnel: w1372 -> [w1378 w1382]
              tunnel: [w1378 w1381] -> w1366
              tunnel: [w1377 w1380] -> w1365
              tunnel: w1371 -> [w1377 w1379]
              frame False {
              }
              frame True {
                n811 = property on="Z Scan Length SP steps" class="DigNum (strict)"() -> ("Value"=w1383:i32)  [unwired: 2 in, 2 out]
                n812 = Number To Decimal String(number=w1383) -> (decimal integer string=w1384:string)  [unwired: 1 in]
                n813 = call "Applied Send Command.vi"("error in (no error)"=w1379, "Extra"=w1384, "Command"=T1."Distance or Position", "VISA resource name"=w1382) -> ("error out"=w1380:errorcluster, "VISA resource name out"=w1381:refnum<visa-resource-name>)  [unwired: 3 in, 1 out]
              }
            }
          }
          frame #1 {
            n814 = case shown="True" w1404 {
              tunnel: w1418 -> [w1434 w1438]
              tunnel: [w1434 w1437] -> w1417
              tunnel: w1416 -> [w1433 w1436]
              tunnel: [w1433 w1435] -> w1415
              frame False {
              }
              frame True {
                n815 = call "Applied Send Command.vi"("error in (no error)"=w1436, "Command"=T1."Feed to Length", "VISA resource name"=w1438) -> ("error out"=w1435:errorcluster, "VISA resource name out"=w1437:refnum<visa-resource-name>)  [unwired: 4 in, 1 out]
              }
            }
            n816 = case shown="True" w1405 {
              tunnel: w1414 -> [w1427 w1431]
              tunnel: [w1427 w1430] -> w1413
              tunnel: w1412 -> [w1426 w1429]
              tunnel: [w1426 w1428] -> w1411
              frame False {
              }
              frame True {
                n817 = call "Applied Send Command.vi"("error in (no error)"=w1429, "Command"=T1."Feed to Length", "VISA resource name"=w1431) -> ("error out"=w1428:errorcluster, "VISA resource name out"=w1430:refnum<visa-resource-name>)  [unwired: 4 in, 1 out]
              }
            }
            n818 = case shown="False" w1406 {
              tunnel: w1410 -> [w1420 w1424]
              tunnel: [w1420 w1423] -> w1409
              tunnel: [w1419 w1422] -> w1408
              tunnel: w1407 -> [w1419 w1421]
              frame False {
              }
              frame True {
                n819 = call "Applied Send Command.vi"("error in (no error)"=w1421, "Command"=T1."Feed to Length", "VISA resource name"=w1424) -> ("error out"=w1422:errorcluster, "VISA resource name out"=w1423:refnum<visa-resource-name>)  [unwired: 4 in, 1 out]
              }
            }
          }
          frame #2 {
            (unwired) FALSE ("Slew Ready 2")
            n820 = call "Time Delay7"("Delay Time (s)"=0.1) -> ()  [unwired: 10 in, 1 out]
            n821 = property on="Z Scan" class="Bool (strict)"("Val(Sgnl)"=FALSE ("Slew Ready 2")) -> ()  [unwired: 2 in, 2 out]
            n822 = property on="X Scan" class="Bool (strict)"("Val(Sgnl)"=FALSE ("Slew Ready 2")) -> ()  [unwired: 2 in, 2 out]
            n823 = property on="Y Scan" class="Bool (strict)"("Val(Sgnl)"=FALSE ("Slew Ready 2")) -> ()  [unwired: 2 in, 2 out]
            n824 = property on="Z Scan Velocity SP steps/sec" class="DigNum (strict)"("DisabledEnum"=T2."Enabled" ("Disabled")) -> ()  [unwired: 2 in, 2 out]
            n825 = property on="X Scan Length SP steps" class="DigNum (strict)"("DisabledEnum"=T2."Enabled" ("Disabled")) -> ()  [unwired: 2 in, 2 out]
            n826 = property on="Y Scan Selocity SP steps/sec" class="DigNum (strict)"("DisabledEnum"=T2."Enabled" ("Disabled")) -> ()  [unwired: 2 in, 2 out]
            n827 = property on="Z Scan Length SP steps" class="DigNum (strict)"("DisabledEnum"=T2."Enabled" ("Disabled")) -> ()  [unwired: 2 in, 2 out]
            n828 = property on="Y Scan Length SP steps" class="DigNum (strict)"("DisabledEnum"=T2."Enabled" ("Disabled")) -> ()  [unwired: 2 in, 2 out]
            n829 = property on="X Scan Velocity SP steps/sec" class="DigNum (strict)"("DisabledEnum"=T2."Enabled" ("Disabled")) -> ()  [unwired: 2 in, 2 out]
            n830 = property on="Scan Go" class="Bool"("DisabledEnum"=T2."Disabled and Grayed Out" ("Disabled")) -> ()  [unwired: 2 in, 2 out]
            n831 = property on="Scan Cancel" class="Bool"("DisabledEnum"=T2."Disabled and Grayed Out" ("Disabled")) -> ()  [unwired: 2 in, 2 out]
          }
        }
      }
      event "Reset": Mouse Down {
        n832 = event-data() -> ()  [unwired: 1 in, 7 out]
        n833 = flat-sequence {
          tunnel: [w1477] -> w1463
          tunnel: w1464 -> [w1479]
          tunnel: [w1478] -> w1462
          tunnel: w1465 -> [w1480]
          frame #0 {
            n834 = property on="Reset X Motor Steps" class="DigNum (strict)"() -> ("Value"=w1483:i32)  [unwired: 2 in, 2 out]
            n835 = Number To Decimal String(number=w1483) -> (decimal integer string=w1481:string)  [unwired: 1 in]
            n836 = call "Applied Send Command.vi"("error in (no error)"=w1479, "Extra"=w1481, "Command"=T1."Set ABS Position", "VISA resource name"=w1480) -> ("error out"=w1478:errorcluster, "VISA resource name out"=w1477:refnum<visa-resource-name>)  [unwired: 3 in, 1 out]
          }
        }
        n837 = flat-sequence {
          tunnel: w1469 -> [w1488]
          tunnel: w1468 -> [w1485]
          tunnel: [w1487] -> w1467
          tunnel: [w1486] -> w1466
          frame #0 {
            n838 = property on="Reset Y Motor Steps" class="DigNum (strict)"() -> ("Value"=w1490:i32)  [unwired: 2 in, 2 out]
            n839 = Number To Decimal String(number=w1490) -> (decimal integer string=w1489:string)  [unwired: 1 in]
            n840 = call "Applied Send Command.vi"("error in (no error)"=w1485, "Extra"=w1489, "Command"=T1."Set ABS Position", "VISA resource name"=w1488) -> ("error out"=w1486:errorcluster, "VISA resource name out"=w1487:refnum<visa-resource-name>)  [unwired: 3 in, 1 out]
          }
        }
        n841 = flat-sequence {
          tunnel: [w1475] -> w1459
          tunnel: [w1474] -> w1458
          tunnel: w1461 -> [w1472]
          tunnel: w1460 -> [w1473]
          frame #0 {
            n842 = property on="Reset Z Motor Steps" class="DigNum (strict)"() -> ("Value"=w1476:i32)  [unwired: 2 in, 2 out]
            n843 = Number To Decimal String(number=w1476) -> (decimal integer string=w1470:string)  [unwired: 1 in]
            n844 = call "Applied Send Command.vi"("error in (no error)"=w1473, "Extra"=w1470, "Command"=T1."Set ABS Position", "VISA resource name"=w1472) -> ("error out"=w1474:errorcluster, "VISA resource name out"=w1475:refnum<visa-resource-name>)  [unwired: 3 in, 1 out]
          }
        }
      }
    }
    n845 = case shown="True" "Delete Button" {
      tunnel: w292 -> [_ w315]
      frame False {
      }
      frame True {
        n846 = property on="Preset positions" class="Ring (strict)"() -> ("Value"=w313:i32)  [unwired: 2 in, 2 out]
        n847 = Delete From Array(array=w315, index=w313) -> (array with subset deleted=w314:string[])  [unwired: 1 in, 1 out]
        n848 = property on="Presets" class="Arr (strict)"() -> ("Value"=w312:i32[][])  [unwired: 2 in, 2 out]
        n849 = property on="Preset positions" class="Ring (strict)"("Strings []"=w314) -> ()  [unwired: 2 in, 2 out]
        n850 = Delete From Array(array=w312, index (row)=w313) -> (array with subset deleted=w311:i32[][])  [unwired: 2 in, 1 out]
        n851 = property on="Presets" class="Arr (strict)"("Val(Sgnl)"=w311) -> ()  [unwired: 2 in, 2 out]
      }
    }
    n852 = Build Array(w288, w287, w286) -> (w285:dbl[])
    n853 = call-poly <userlib>:"CaLabPut.vi"("Values"=w285, "PV Names"=string[] ["SSE:TmtX", "SSE:TmtY", "SSE:TmtZ"]) -> ()  [unwired: 6 in, 4 out]
    n854 = case shown="True" "Set Button" {
      tunnel: "Preset positions" -> [_ w331]
      frame False {
      }
      frame True {
        n855 = property on="Presets" class="Arr (strict)"() -> ("Value"=w328:i32[][])  [unwired: 2 in, 2 out]
        n856 = Index Array(array=w328, index (row)=w331) -> (element=w330:i32[])  [unwired: 1 in]
        n857 = Array To Cluster(array=w330) -> (cluster=w329:T4)
        n858 = Unbundle(w329) -> ("Value[0]"=w327:i32, "Value[1]"=w326:i32, "Value[2]"=w325:i32)  [unwired: 6 out]
        n859 = property on="X Step SP" class="DigNum (strict)"("Val(Sgnl)"=w327) -> ()  [unwired: 2 in, 2 out]
        n860 = property on="Y Step SP" class="DigNum (strict)"("Val(Sgnl)"=w326) -> ()  [unwired: 2 in, 2 out]
        n861 = property on="Z Step SP" class="DigNum (strict)"("Val(Sgnl)"=w325) -> ()  [unwired: 2 in, 2 out]
      }
    }
    n862 = case shown="True" "Add Button" {
      tunnel: w292 -> [_ w324]
      frame False {
      }
      frame True {
        n863 = property on="X Step PV" class="DigNum (strict)"() -> ("Value"=w319:i32)  [unwired: 2 in, 2 out]
        n864 = property on="Y Step PV" class="DigNum (strict)"() -> ("Value"=w318:i32)  [unwired: 2 in, 2 out]
        n865 = property on="Z Step PV" class="DigNum (strict)"() -> ("Value"=w317:i32)  [unwired: 2 in, 2 out]
        n866 = Build Array(w319, w318, w317) -> (w322:i32[])
        n867 = Build Array (concatenate)(w324, "String") -> (w323:string[])
        n868 = property on="Preset positions" class="Ring (strict)"("Strings []"=w323) -> ()  [unwired: 2 in, 2 out]
        n869 = property on="Presets" class="Arr (strict)"() -> ("Value"=w321:i32[][])  [unwired: 2 in, 2 out]
        n870 = Build Array (concatenate)(w321, w322) -> (w316:i32[][])
        n871 = property on="Presets" class="Arr (strict)"("Val(Sgnl)"=w316) -> ()  [unwired: 2 in, 2 out]
      }
    }
  }
  n872 = flat-sequence {
    tunnel: w55 -> [w1492]
    tunnel: w54 -> [w1491]
    tunnel: [w1503] -> w39
    frame #0 {
      # "GET CURRENT POSITION"
      n873 = call "Applied Send Command.vi"("error in (no error)"=w1491, "Extra"="", "Command"=T1."Immediate Position?", "VISA resource name"=w1492) -> ("error out"=w1493:errorcluster, "read buffer"=w1498:string, "VISA resource name out"=w1494:refnum<visa-resource-name>)  [unwired: 3 in]
      n874 = call "Applied Send Command.vi"("error in (no error)"=w1493, "Command"=T1."Stop & Kill Buffer", "VISA resource name"=w1494) -> ("error out"=w1500:errorcluster, "VISA resource name out"=w1501:refnum<visa-resource-name>)  [unwired: 4 in, 1 out]
      n875 = Hexadecimal String To Number(string=w1498, offset=3) -> (number=w1495:u32)  [unwired: 1 in, 1 out]
      n876 = VISA Close(VISA resource name=w1501, error in (no error)=w1500) -> ()  [unwired: 1 out]
      n877 = To Long Integer(number=w1495) -> (32bit integer=w1503:i32)
    }
  }
  n878 = flat-sequence {
    tunnel: w41 -> [w1506]
    tunnel: w40 -> [w1505]
    tunnel: [w1504] -> w38
    frame #0 {
      # "GET CURRENT POSITION"
      n879 = call "Applied Send Command.vi"("error in (no error)"=w1505, "Extra"="", "Command"=T1."Immediate Position?", "VISA resource name"=w1506) -> ("error out"=w1507:errorcluster, "read buffer"=w1512:string, "VISA resource name out"=w1508:refnum<visa-resource-name>)  [unwired: 3 in]
      n880 = call "Applied Send Command.vi"("error in (no error)"=w1507, "Command"=T1."Stop & Kill Buffer", "VISA resource name"=w1508) -> ("error out"=w1514:errorcluster, "VISA resource name out"=w1515:refnum<visa-resource-name>)  [unwired: 4 in, 1 out]
      n881 = Hexadecimal String To Number(string=w1512, offset=3) -> (number=w1509:u32)  [unwired: 1 in, 1 out]
      n882 = VISA Close(VISA resource name=w1515, error in (no error)=w1514) -> ()  [unwired: 1 out]
      n883 = To Long Integer(number=w1509) -> (32bit integer=w1504:i32)
    }
  }
  n884 = flat-sequence {
    tunnel: w43 -> [w1518]
    tunnel: w42 -> [w1517]
    tunnel: [w1519] -> w37
    frame #0 {
      # "GET CURRENT POSITION"
      n885 = call "Applied Send Command.vi"("error in (no error)"=w1517, "Extra"="", "Command"=T1."Immediate Position?", "VISA resource name"=w1518) -> ("error out"=w1520:errorcluster, "read buffer"=w1525:string, "VISA resource name out"=w1521:refnum<visa-resource-name>)  [unwired: 3 in]
      n886 = call "Applied Send Command.vi"("error in (no error)"=w1520, "Command"=T1."Stop & Kill Buffer", "VISA resource name"=w1521) -> ("error out"=w1527:errorcluster, "VISA resource name out"=w1528:refnum<visa-resource-name>)  [unwired: 4 in, 1 out]
      n887 = Hexadecimal String To Number(string=w1525, offset=3) -> (number=w1522:u32)  [unwired: 1 in, 1 out]
      n888 = VISA Close(VISA resource name=w1528, error in (no error)=w1527) -> ()  [unwired: 1 out]
      n889 = To Long Integer(number=w1522) -> (32bit integer=w1519:i32)
    }
  }
  n890 = flat-sequence {
    tunnel: w39 -> [w1534]
    tunnel: w38 -> [w1533]
    tunnel: w37 -> [w1532]
    frame #0 {
      n891 = Build Array(w1534, w1533, w1532) -> (w1530:i32[])
      n892 = call-poly <vilib>:"Write To Spreadsheet File.vi"("1D data"=w1530, "file path (dialog if empty)"=path "S:/SSE/SCL2/POS.TXT") -> ()  [unwired: 6 in, 1 out]
    }
    frame #1 {
      n893 = property on="Presets" class="Arr (strict)"() -> ("Value"=w1541:i32[][])  [unwired: 2 in, 2 out]
      n894 = property on="Preset positions" class="Ring (strict)"() -> ("Strings []"=w1537:string[])  [unwired: 2 in, 2 out]
      n895 = Number To Decimal String(number=w1541) -> (decimal integer string=w1535:string[][])  [unwired: 1 in]
      n896 = Transpose 2D Array(2D array=w1535) -> (transposed array=w1536:string[][])
      n897 = Build Array (concatenate)(w1537, w1536) -> (w1538:string[][])
      n898 = Transpose 2D Array(2D array=w1538) -> (transposed array=w1539:string[][])
      n899 = call-poly <vilib>:"Write To Spreadsheet File.vi"("2D data"=w1539, "file path (dialog if empty)"=path "S:/SSE/SCL2/PRESET.TXT") -> ()  [unwired: 6 in, 1 out]
    }
  }
